vi "PointGrey Grasshopper_Cam_BACKUP.vi"(0 "Operation":T2(ring), 1 "Camera-specific in":variant, 5 "Exposure time (s)":dbl, 7 "Save path":path, 9 "Capture mode":enum16{"Single frame", "Sequence"}(ring), 11 "Capture button":refnum<vi>, 12 "Image in":variant, 14 "Frames in sequence":u32) -> (3 "Camera-specific out":variant, 4 "Status":T1)   [LabVIEW 2015]
uses:
  <vilib>/userdefined/High Color/IMAQdx.ctl
  <vilib>/vision/Image Controls.llb/IMAQ Image.ctl
  <vilib>/vision/driver/IMAQdx.llb/IMAQdx Camera Control Mode.ctl
  <vilib>/vision/driver/IMAQdx.llb/IMAQdx Acquisition Mode.ctl
  <vilib>/Platform/TimedLoop/XDataNode/timing_clust.ctl
  <vilib>/Platform/TimedLoop/XDataNode/nitl_modes.ctl
  <vilib>/Platform/TimedLoop/XDataNode/wakeup.ctl
  <vilib>/vision/driver/IMAQdx.llb/IMAQdx Buffer Number Mode.ctl
  <vilib>/platform/TimedLoop/XDataNode/XDataNode.xnode
  <vilib>/vision/driver/NI_Vision_Acquisition_Software.lvlib
  <resource>/objmgr/imaqdx.rc
  <vilib>/Platform/TimedLoop/XDataNode/XDNodeRunTimeDep.lvlib
  <vilib>/vision/NI_Vision_Development_Module.lvlib
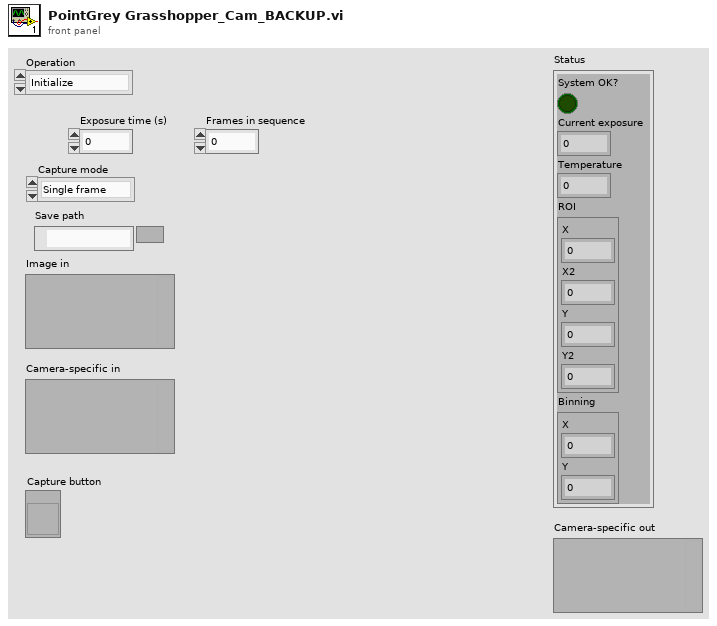
[diagram p1: front panel]
types:
  T1 = cluster{"System OK?":bool, "Current exposure":dbl, "Temperature":dbl, "ROI":cluster{"X":u32, "X2":u32, "Y":u32, "Y2":u32}, "Binning":cluster{"X":u32, "Y":u32}}
  T2 = enum16{"Initialize", "Shut down", "Set capture mode", "Set exposure", "Trigger and read", "Get status", "Other settings"}
  T3 = typedef "IMAQdx.ctl" = refnum<k21>
  T4 = typedef "IMAQ Image.ctl" = refnum<image>
  T5 = typedef "Semaphore RefNum" = refnum<k1>
  T6 = cluster{"Frames to capture":u32, "Current camera":i32, "Camera References":T3[], "Which cameras record":bool[], "Camera event refnums":refnum<event-registration>[], "Image buffers":T4[], "File write access":T5, "Offset and gain":dbl[][], "RGB Channels":enum16{"None", "Camera 1", "Camera 2", "Camera 3"}[], "RGB buffers":T4[], "Camera orientation":enum16{"No rotation, No flip", "No rotation, Flip UD", "No rotation, Flip LR", "Clockwise, No flip", "Clockwise, Flip UD", "Clockwise, Flip LR", "Anticlockwise, No flip", "Anticlockwise, Flip UD", "Anticlockwise, Flip LR"}[]}
  T7 = enum32{"Continuous", "Single frame", "Multi frame"}
  T8 = typedef "NI_Vision_Acquisition_Software.lvlib/IMAQdx Camera Control Mode.ctl" = enum32{"Controller", "Listener"}
  T9 = cluster{"New Image":T4, "Image":refnum<vi>, "FPS target":dbl}
  T10 = enum16{"open", "replace", "create", "open or create", "replace or create", "replace or create with confirmation"}
  T11 = cluster{"File refnum":refnum<file>, "Image File Directory":cluster{cluster{"Field":u16, "Type":u16, "Count":u32, "Value / Offset":u32, "Add IFD Offset?":bool}[], cluster{"Data":u32[], "Add offset?":bool}[]}, "Big endian?":bool, "IFD Offset Size":u32}
  T12 = typedef "NI_Vision_Acquisition_Software.lvlib/IMAQdx Acquisition Mode.ctl" = enum32{"One Shot", "Continuous"}
  T13 = typedef "XDNodeRunTimeDep.lvlib/timing_clust.ctl" = cluster{"Expected End [f-1]":u64, "Actual End [f-1]":u64, "Finished Late? [f-1]":bool, "Expected End [i-1]":u64, "Actual End [i-1]":u64, "Finished Late? [i-1]":bool, "Expected Start [i]":u64, "Actual Start [i]":u64, "Expected Start [f]":u64, "Actual Start [f]":u64, "Source Name":string, "Structure Name":string, "Period":i64, "Deadline":i64, "Offset":i64, "Start":i64, "Priority":i32, "Timeout":i32, "Mode":T14, "Wakeup Reason":T15, "Error":errorcluster, "Source Type":string, "Secondary Source Type":string, "Global End Time":u64, "Global Start Time":u64, "Frame Duration":u64, "Iteration Duration":u64, "Assigned CPU":i32, "I/O Scan Engine Mode":u32}
  T14 = typedef "XDNodeRunTimeDep.lvlib/nitl_modes.ctl" = enum32{"No Change", "Process missed periods, maintain original phase", "Discard missed periods, maintain original phase", "Process missed periods, ignore original phase", "Discard missed periods, ignore original phase"}
  T15 = typedef "XDNodeRunTimeDep.lvlib/wakeup.ctl" = enum32{"Normal", "Aborted", "Asynchronous wakeup", "Timing source error", "Timed loop error", "Timeout"}
  T16 = typedef "NI_Vision_Acquisition_Software.lvlib/IMAQdx Buffer Number Mode.ctl" = enum32{"Next", "Last", "Buffer Number", "Every", "Last New"}
  T17 = enum16{"No rotation, No flip", "No rotation, Flip UD", "No rotation, Flip LR", "Clockwise, No flip", "Clockwise, Flip UD", "Clockwise, Flip LR", "Anticlockwise, No flip", "Anticlockwise, Flip UD", "Anticlockwise, Flip LR"}[]
  T18 = typedef "Image Type" = u32
  T19 = enum16{"None", "Camera 1", "Camera 2", "Camera 3"}[]
  T20 = cluster{"Type":u32, "Version":u32, "Flags":u32, "SerialNumberHigh":u32, "SerialNumberLow":u32, "BusType":u32, "InterfaceName":string, "VendorName":string, "ModelName":string, "CameraFileName":string, "CameraAttributeURL":string}[]
  T21 = enum16{"None", "Camera 1", "Camera 2", "Camera 3"}
  T22 = enum16{"No rotation, No flip", "No rotation, Flip UD", "No rotation, Flip LR", "Clockwise, No flip", "Clockwise, Flip UD", "Clockwise, Flip LR", "Anticlockwise, No flip", "Anticlockwise, Flip UD", "Anticlockwise, Flip LR"}
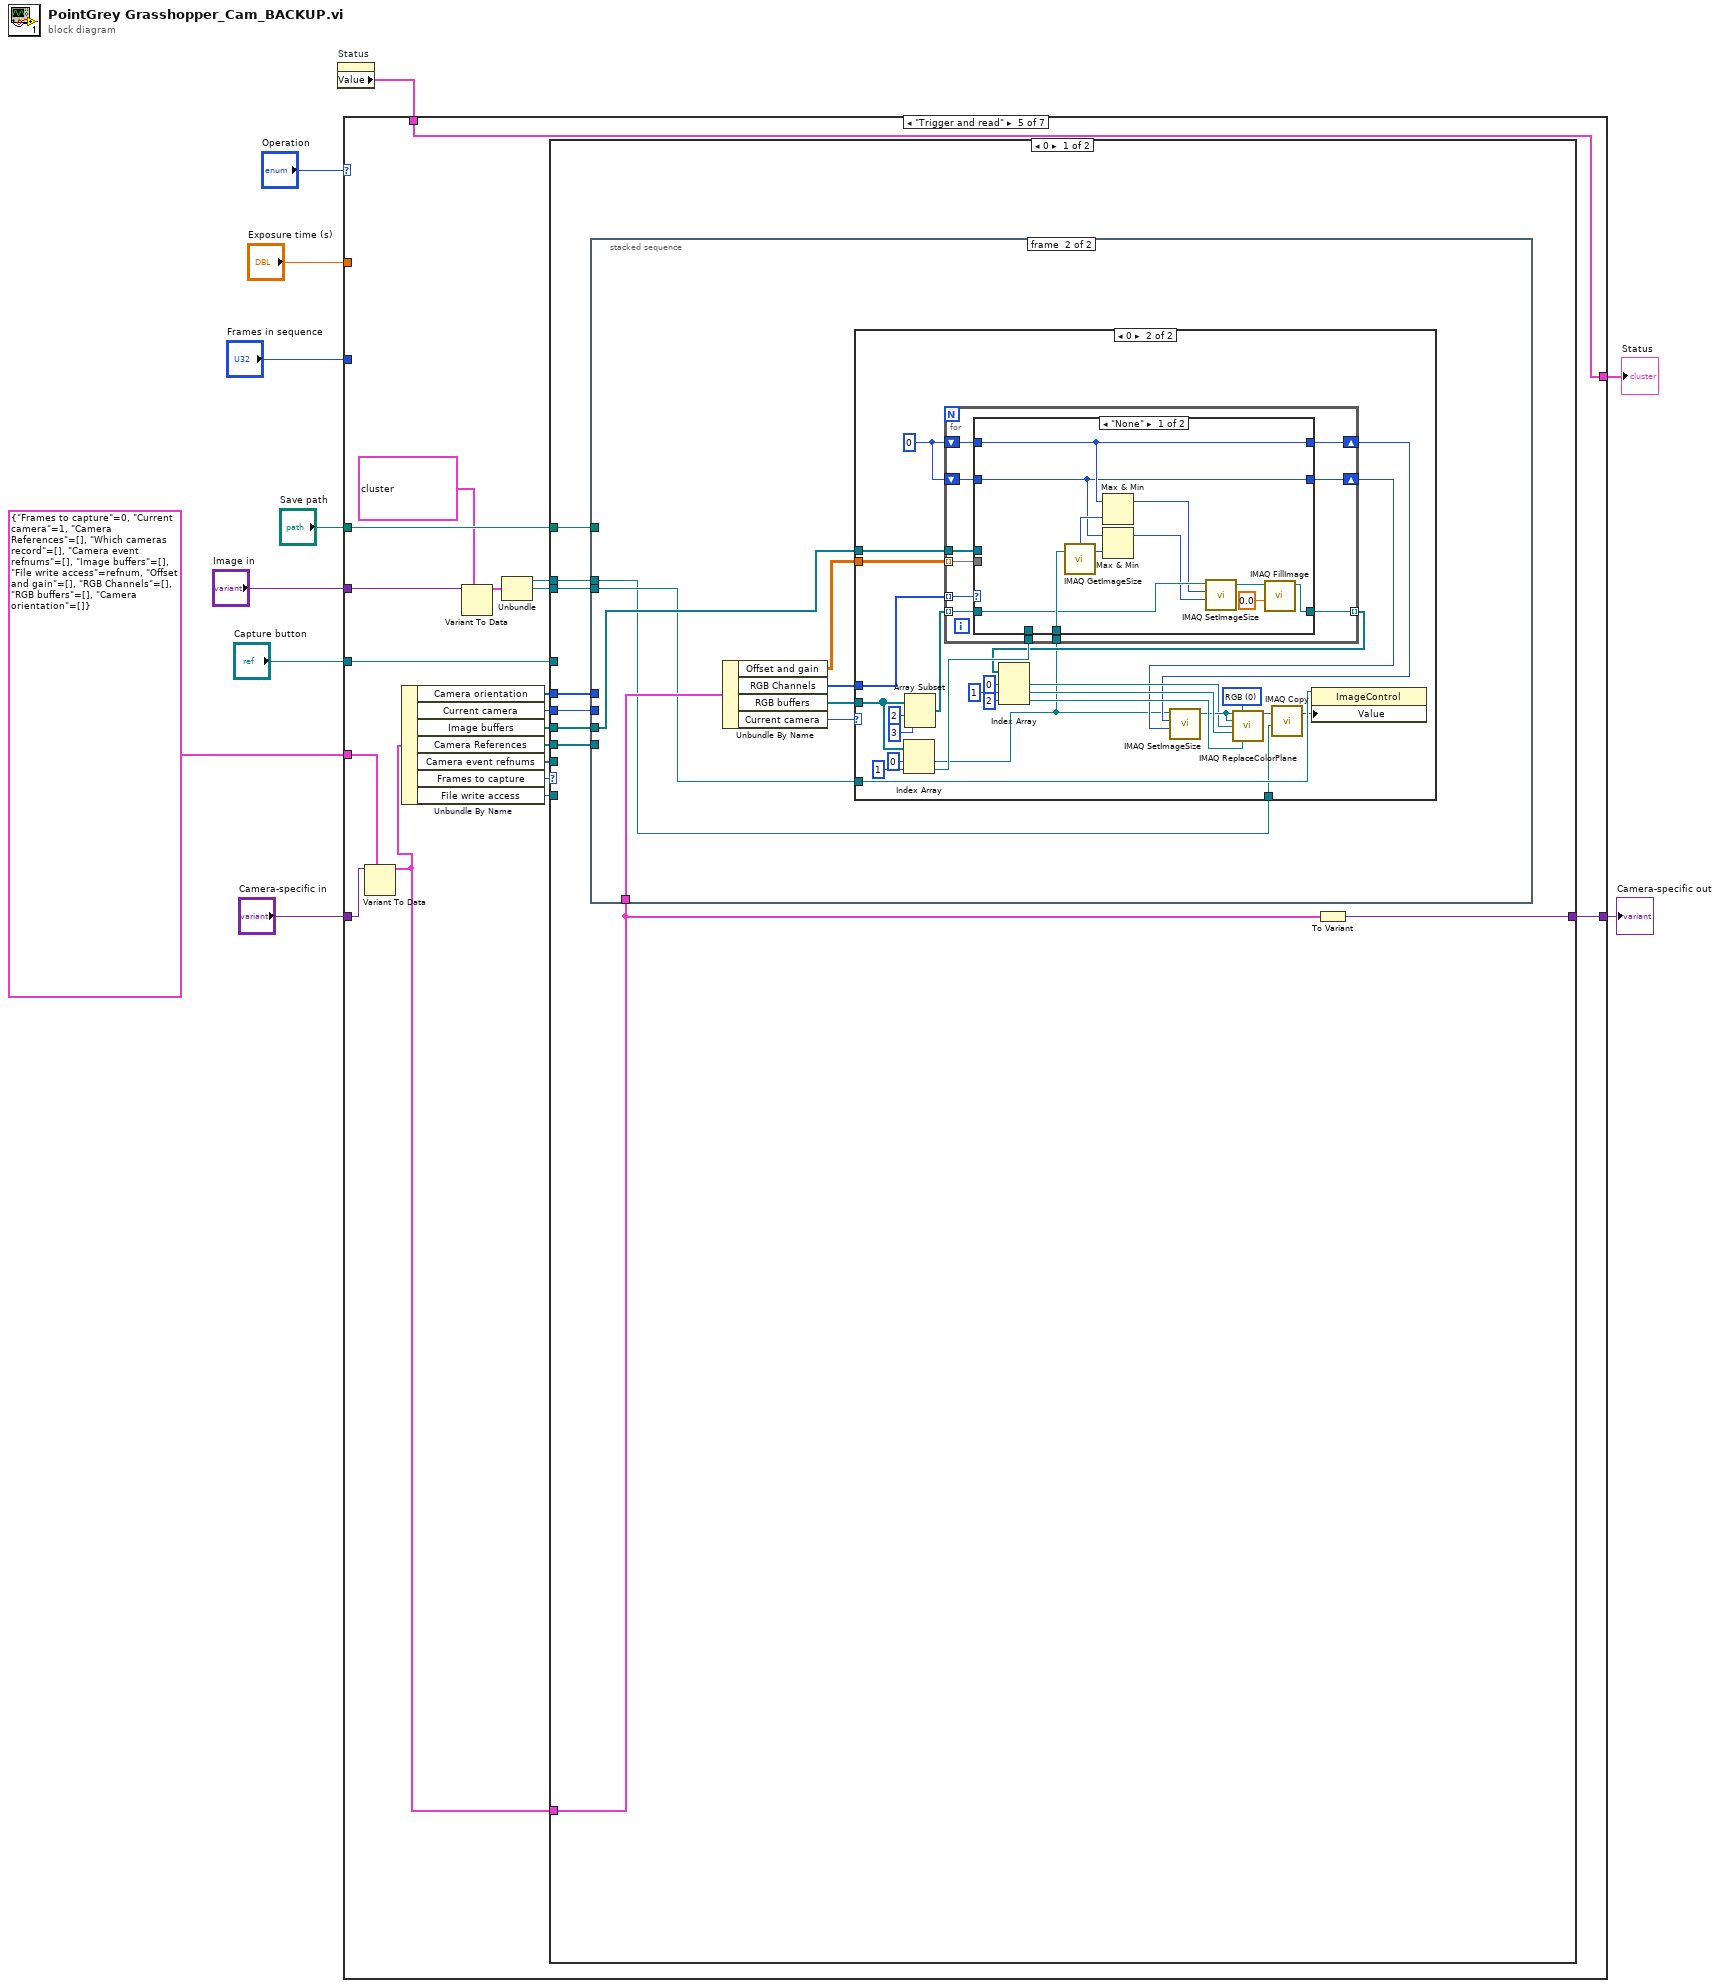
[diagram p0: block diagram]
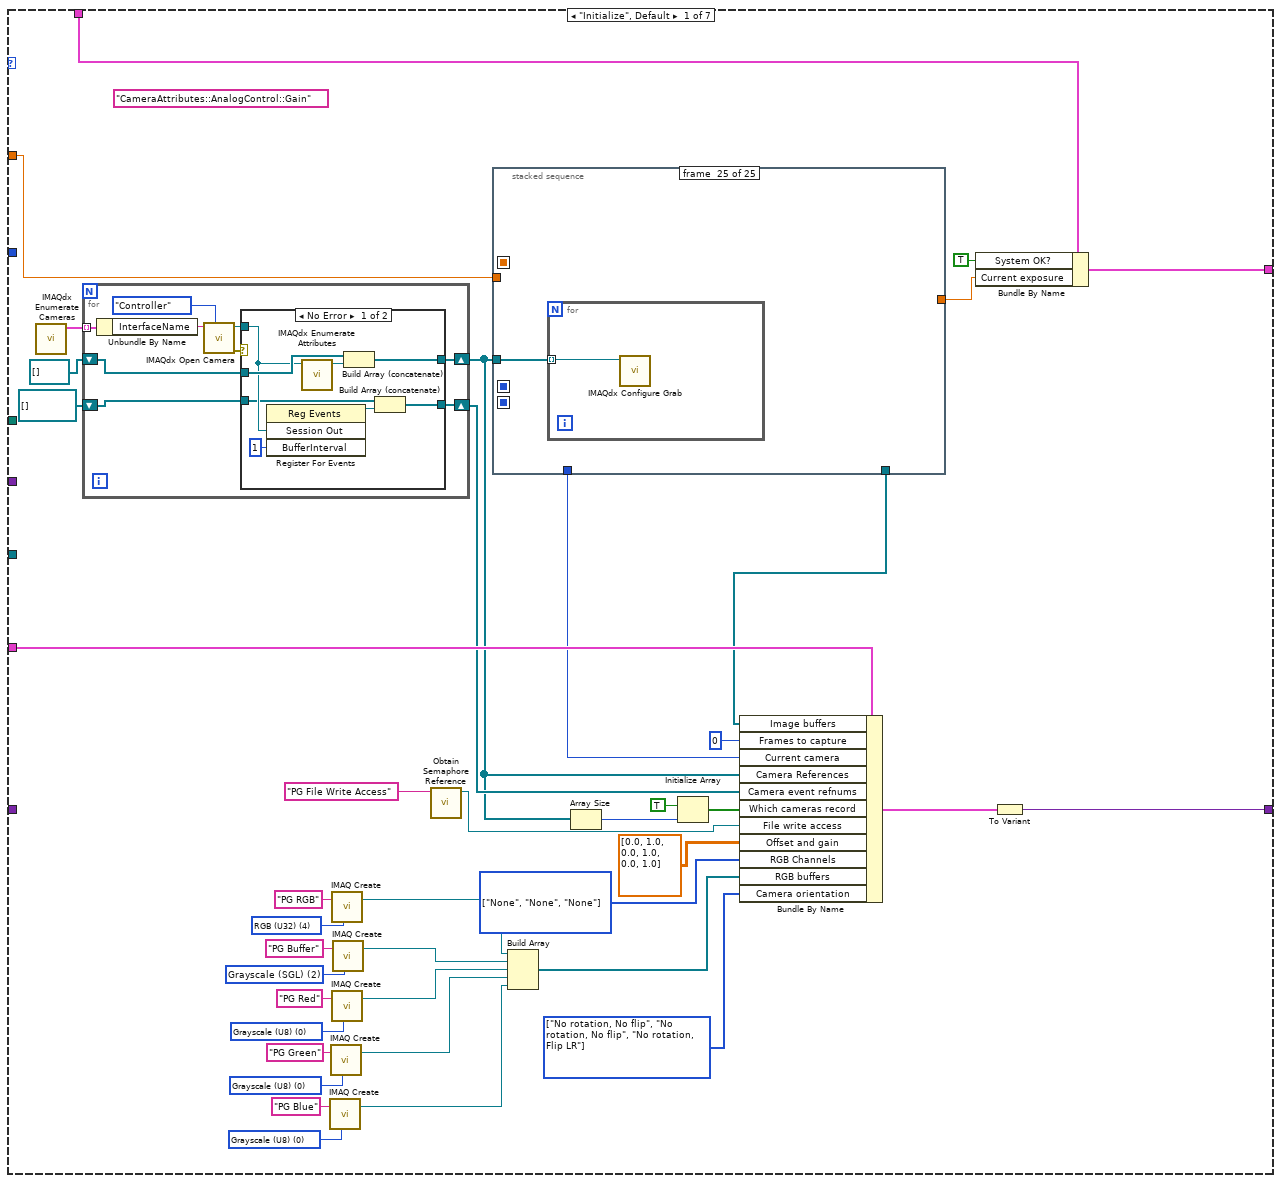
[diagram p2: hidden frame]
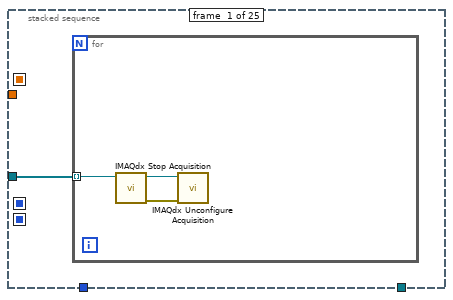
[diagram p3: hidden frame]
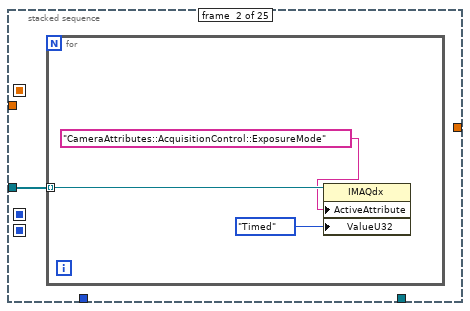
[diagram p4: hidden frame]
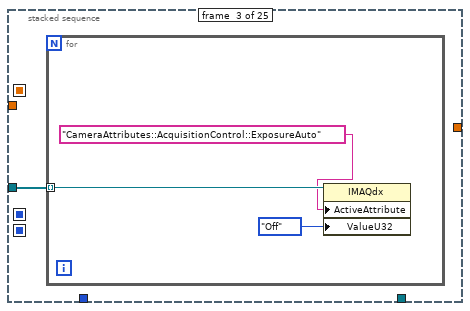
[diagram p5: hidden frame]
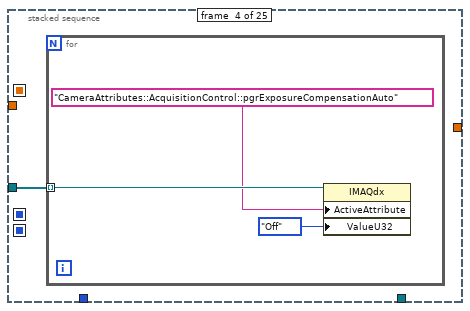
[diagram p6: hidden frame]
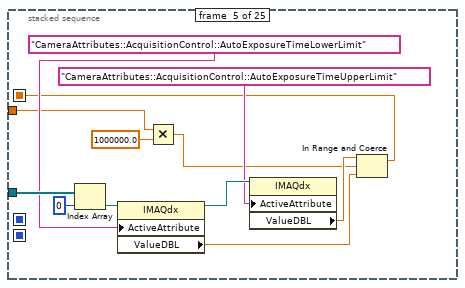
[diagram p7: hidden frame]
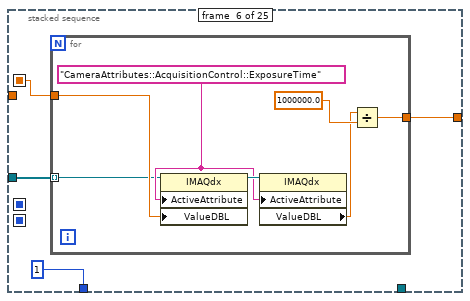
[diagram p8: hidden frame]
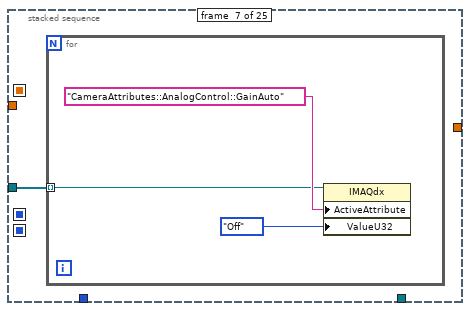
[diagram p9: hidden frame]
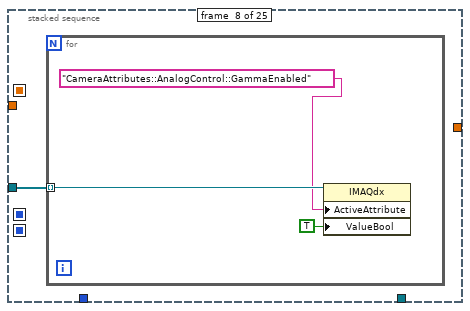
[diagram p10: hidden frame]
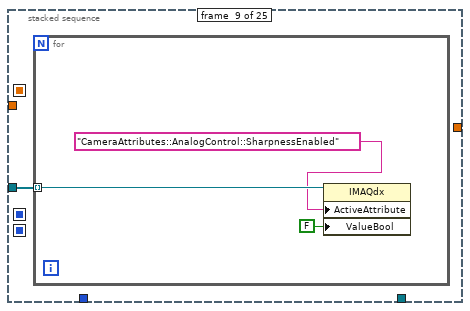
[diagram p11: hidden frame]
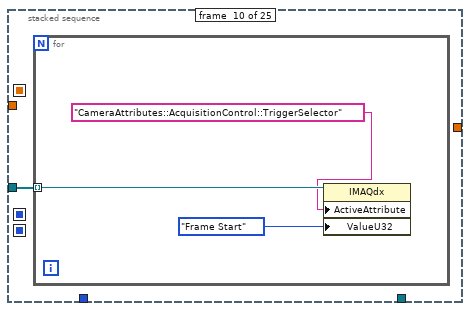
[diagram p12: hidden frame]
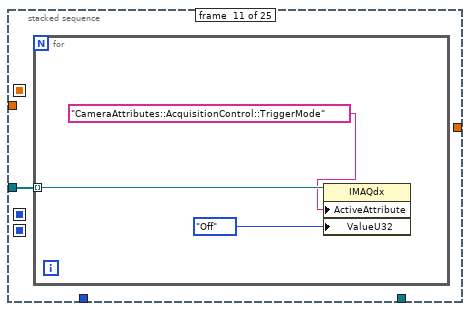
[diagram p13: hidden frame]
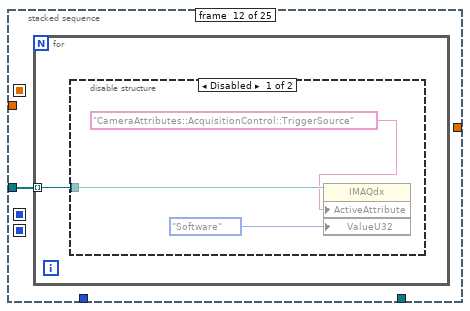
[diagram p14: hidden frame]
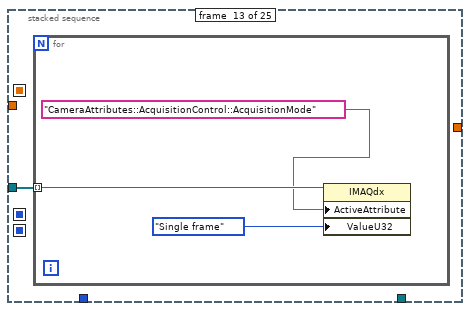
[diagram p16: hidden frame]
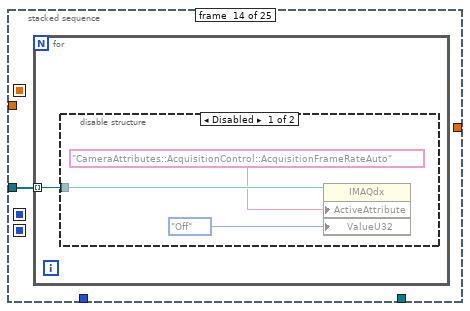
[diagram p17: hidden frame]
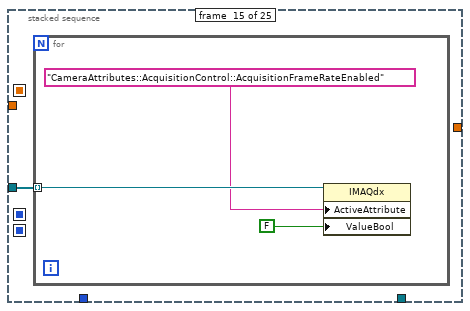
[diagram p19: hidden frame]
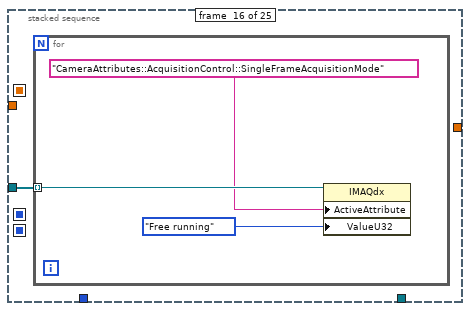
[diagram p20: hidden frame]
diagram:
  n1 = property on="Status" class="Clust (strict)"() -> ("Value"=w9:T1)  [unwired: 2 in, 2 out]
  n2 = case shown="\"Trigger and read\"" "Operation" {
    tunnel: "Exposure time (s)" -> [w40 _ _ w371 _ _ _]
    tunnel: w9 -> [w51 w210 w234 w377 w424 w1366 w1384]
    tunnel: [w50 w210 w234 w376 w424 w1365 w1384] -> w8
    tunnel: "Save path" -> [_ _ _ _ w423 _ _]
    tunnel: "Image in" -> [_ _ _ _ w414 _ _]
    tunnel: [w48 w205 w230 w374 w407 w1362 w1376] -> w5
    tunnel: "Camera-specific in" -> [_ w209 w232 w374 w410 w1362 w1383]
    tunnel: T6 {"Frames to capture"=0, "Current camera"=1, "Camera References"=[], "Which cameras record"=[], "Camera event refnums"=[], "Image buffers"=[], "File write access"=refnum, "Offset and gain"=[], "RGB Channels"=[], "RGB buffers"=[], "Camera orientation"=[]} -> [w49 w204 w231 w375 w422 w1361 w1382]
    tunnel: "Frames in sequence" -> [_ _ w227 _ _ _ _]
    tunnel: "Capture button" -> [_ _ _ _ w406 _ _]
    frame "Initialize", Default {
      w12 = T17 [enum."No rotation, No flip", enum."No rotation, No flip", enum."No rotation, Flip LR"] items=["No rotation, No flip", "No rotation, Flip UD", "No rotation, Flip LR", "Clockwise, No flip", "Clockwise, Flip UD", "Clockwise, Flip LR", "Anticlockwise, No flip", "Anticlockwise, Flip UD", "Anticlockwise, Flip LR"] ("Camera orientation")
      w19 = T18 0 items=["Grayscale (U8)", "Grayscale (I16)", "Grayscale (SGL)", "Complex (CSG)", "RGB (U32)", "HSL (U32)", "RGB (U64)", "Grayscale (U16)"] ("Image Type")
      w20 = T18 0 items=["Grayscale (U8)", "Grayscale (I16)", "Grayscale (SGL)", "Complex (CSG)", "RGB (U32)", "HSL (U32)", "RGB (U64)", "Grayscale (U16)"] ("Image Type")
      w21 = T18 0 items=["Grayscale (U8)", "Grayscale (I16)", "Grayscale (SGL)", "Complex (CSG)", "RGB (U32)", "HSL (U32)", "RGB (U64)", "Grayscale (U16)"] ("Image Type")
      w22 = T18 2 items=["Grayscale (U8)", "Grayscale (I16)", "Grayscale (SGL)", "Complex (CSG)", "RGB (U32)", "HSL (U32)", "RGB (U64)", "Grayscale (U16)"] ("Image Type")
      w23 = T18 4 items=["Grayscale (U8)", "Grayscale (I16)", "Grayscale (SGL)", "Complex (CSG)", "RGB (U32)", "HSL (U32)", "RGB (U64)", "Grayscale (U16)"] ("Image Type")
      w29 = T19 [enum."None", enum."None", enum."None"] items=["None", "Camera 1", "Camera 2", "Camera 3"] ("RGB Channels")
      (unwired) "CameraAttributes::AnalogControl::Gain"
      n3 = call <vilib>:"IMAQdx Enumerate Cameras.vi"() -> ("Camera Information Array"=w46:T20)  [unwired: 10 in, 1 out]
      n4 = for {
        tunnel: w46 -> [w190] mode=indexing
        shift-right: [w185] -> w38
        shift-left: T3[] [] -> [w183]
        shift-right: [w186] -> w43
        shift-left: refnum<event-registration>[] [] -> [w182]
        n5 = Unbundle By Name(w190) -> ("InterfaceName"=w189:string)
        n6 = call <vilib>:"IMAQdx Open Camera.vi"("Camera Control Mode"=IMAQdx_Camera_Control_Mode."Controller", "Session In"=w189) -> ("error out"=w184:errorcluster, "Session Out"=w187:T3)  [unwired: 8 in]
        n7 = case shown="No Error" w184 {
          tunnel: w187 -> [w194 _]
          tunnel: [w193 w199] -> w186
          tunnel: [w196 w200] -> w185
          tunnel: w183 -> [w195 w200]
          tunnel: w182 -> [w191 w199]
          frame No Error {
            n8 = register-events(w194, u32 1 ("BufferInterval")) -> (reference out=w192:refnum<event-registration>)  [unwired: 2 in, 1 out]
            n9 = call <vilib>:"IMAQdx Enumerate Attributes.vi"("Session In"=w194) -> ("Session Out"=w197:T3)  [unwired: 8 in, 2 out]
            n10 = Build Array (concatenate)(w195, w197) -> (w196:T3[])
            n11 = Build Array (concatenate)(w191, w192) -> (w193:refnum<event-registration>[])
          }
          frame Error {
          }
        }
      }
      n12 = call "IMAQ Create"("Image Name"="PG Blue", "Image Type"=w19) -> ("New Image"=w14:T4)  [unwired: 3 in, 1 out]
      n13 = call "IMAQ Create"("Image Name"="PG Green", "Image Type"=w20) -> ("New Image"=w15:T4)  [unwired: 3 in, 1 out]
      n14 = call "IMAQ Create"("Image Name"="PG RGB", "Image Type"=w23) -> ("New Image"=w18:T4)  [unwired: 3 in, 1 out]
      n15 = call "IMAQ Create"("Image Name"="PG Red", "Image Type"=w21) -> ("New Image"=w16:T4)  [unwired: 3 in, 1 out]
      n16 = call "IMAQ Create"("Image Name"="PG Buffer", "Image Type"=w22) -> ("New Image"=w17:T4)  [unwired: 3 in, 1 out]
      n17 = call <vilib>:"Obtain Semaphore Reference.vi"("name (unnamed)"="PG File Write Access") -> ("semaphore"=w31:T5)  [unwired: 4 in, 2 out]
      n18 = stacked-sequence {
        seq-local: [_ _ _ _ w71 _ _ _ _ _ _ _ _ _ _ _ _ _ _ _ _ _ _ _ _] -> [_ _ _ _ _ w80 _ _ _ _ _ _ _ _ _ _ _ _ _ _ _ _ _ _ _]
        seq-local: [_ _ _ _ _ _ _ _ _ _ _ _ _ _ _ _ _ w137 _ _ _ _ _ _ _] -> [_ _ _ _ _ _ _ _ _ _ _ _ _ _ _ _ _ _ _ _ _ _ _ w167 _]
        seq-local: [_ _ _ _ _ _ _ _ _ _ _ _ _ _ _ _ _ _ w143 _ _ _ _ _ _] -> [_ _ _ _ _ _ _ _ _ _ _ _ _ _ _ _ _ _ _ _ _ _ _ w166 _]
        tunnel: w38 -> [w52 w56 w60 w64 w77 w83 w91 w95 w99 w103 w107 w111 w116 w120 w125 w129 w133 w138 w144 w149 w153 w157 w161 w168 w180]
        tunnel: [_ _ _ _ _ 1 ("index") _ _ _ _ _ _ _ _ _ _ _ _ _ _ _ _ _ _ _] -> w41
        tunnel: w40 -> [_ _ _ _ w69 _ _ _ _ _ _ _ _ _ _ _ _ _ _ _ _ _ _ _ _]
        tunnel: [_ _ _ _ _ w81 _ _ _ _ _ _ _ _ _ _ _ _ _ _ _ _ _ _ _] -> w39
        tunnel: [_ _ _ _ _ _ _ _ _ _ _ _ _ _ _ _ _ _ _ _ _ _ _ w165 _] -> w34
        frame #0 {
          n19 = for {
            tunnel: w52 -> [w55] mode=indexing
            n20 = call <vilib>:"IMAQdx Stop Acquisition.vi"("Session In"=w55) -> ("error out"=w53:errorcluster, "Session Out"=w54:T3)  [unwired: 9 in]
            n21 = call <vilib>:"IMAQdx Unconfigure Acquisition.vi"("error in"=w53, "Session In"=w54) -> ()  [unwired: 8 in, 2 out]
          }
        }
        frame #1 {
          n22 = for {
            tunnel: w56 -> [w59] mode=indexing
            n23 = property class="IMAQdx"(reference=w59, "ActiveAttribute"="CameraAttributes::AcquisitionControl::ExposureMode", "ValueU32"=enum32{"Timed", "Trigger Width"}."Timed") -> ()  [unwired: 1 in, 2 out]
          }
        }
        frame #2 {
          n24 = for {
            tunnel: w60 -> [w63] mode=indexing
            n25 = property class="IMAQdx"(reference=w63, "ActiveAttribute"="CameraAttributes::AcquisitionControl::ExposureAuto", "ValueU32"=enum32{"Off", "Once", "Continuous"}."Off") -> ()  [unwired: 1 in, 2 out]
          }
        }
        frame #3 {
          n26 = for {
            tunnel: w64 -> [w67] mode=indexing
            n27 = property class="IMAQdx"(reference=w67, "ActiveAttribute"="CameraAttributes::AcquisitionControl::pgrExposureCompensationAuto", "ValueU32"=enum32{"Off", "Once", "Continuous"}."Off") -> ()  [unwired: 1 in, 2 out]
          }
        }
        frame #4 {
          n28 = Index Array(array=w77, index=0) -> (element=w79:T3)
          n29 = property class="IMAQdx"(reference=w79, "ActiveAttribute"="CameraAttributes::AcquisitionControl::AutoExposureTimeLowerLimit") -> (reference out=w75:T3, "ValueDBL"=w73:dbl)  [unwired: 1 in, 1 out]
          n30 = Multiply(x=w69, y=1000000.0) -> (x*y=w68:dbl)
          n31 = property class="IMAQdx"(reference=w75, "ActiveAttribute"="CameraAttributes::AcquisitionControl::AutoExposureTimeUpperLimit") -> ("ValueDBL"=w72:dbl)  [unwired: 1 in, 2 out]
          n32 = In Range and Coerce(upper limit=w72, x=w68, lower limit=w73) -> (coerced(x)=w71:dbl)  [unwired: 1 out]
        }
        frame #5 {
          n33 = for {
            tunnel: w83 -> [w84] mode=indexing
            tunnel: [w87] -> w81
            tunnel: w80 -> [w85]
            w86 = "CameraAttributes::AcquisitionControl::ExposureTime"
            n34 = property class="IMAQdx"(reference=w84, "ActiveAttribute"=w86, "ValueDBL"=w85) -> (reference out=w90:T3)  [unwired: 1 in, 1 out]
            n35 = property class="IMAQdx"(reference=w90, "ActiveAttribute"=w86) -> ("ValueDBL"=w88:dbl)  [unwired: 1 in, 2 out]
            n36 = Divide(x=w88, y=1000000.0) -> (x/y=w87:dbl)
          }
        }
        frame #6 {
          n37 = for {
            tunnel: w91 -> [w92] mode=indexing
            n38 = property class="IMAQdx"(reference=w92, "ActiveAttribute"="CameraAttributes::AnalogControl::GainAuto", "ValueU32"=enum32{"Off", "Once", "Continuous"}."Off") -> ()  [unwired: 1 in, 2 out]
          }
        }
        frame #7 {
          n39 = for {
            tunnel: w95 -> [w98] mode=indexing
            n40 = property class="IMAQdx"(reference=w98, "ActiveAttribute"="CameraAttributes::AnalogControl::GammaEnabled", "ValueBool"=TRUE) -> ()  [unwired: 1 in, 2 out]
          }
        }
        frame #8 {
          n41 = for {
            tunnel: w99 -> [w102] mode=indexing
            n42 = property class="IMAQdx"(reference=w102, "ActiveAttribute"="CameraAttributes::AnalogControl::SharpnessEnabled", "ValueBool"=FALSE) -> ()  [unwired: 1 in, 2 out]
          }
        }
        frame #9 {
          n43 = for {
            tunnel: w103 -> [w106] mode=indexing
            n44 = property class="IMAQdx"(reference=w106, "ActiveAttribute"="CameraAttributes::AcquisitionControl::TriggerSelector", "ValueU32"=enum32{"Frame Start", "Exposure Active"}."Frame Start") -> ()  [unwired: 1 in, 2 out]
          }
        }
        frame #10 {
          n45 = for {
            tunnel: w107 -> [w110] mode=indexing
            n46 = property class="IMAQdx"(reference=w110, "ActiveAttribute"="CameraAttributes::AcquisitionControl::TriggerMode", "ValueU32"=enum32{"Off", "On"}."Off") -> ()  [unwired: 1 in, 2 out]
          }
        }
        frame #11 {
          n47 = for {
            tunnel: w111 -> [w112] mode=indexing
            n48 = disable-structure shown="Disabled" {
              disable-tunnel: w112 -> [w115 _]
              frame Disabled {
                n49 = property class="IMAQdx"(reference=w115, "ActiveAttribute"="CameraAttributes::AcquisitionControl::TriggerSource", "ValueU32"=enum32{"Software", "Line 0", "Line 2", "Line 3"}."Software") -> ()  [unwired: 1 in, 2 out]
              }
              frame Enabled {
              }
            }
          }
        }
        frame #12 {
          n50 = for {
            tunnel: w116 -> [w119] mode=indexing
            n51 = property class="IMAQdx"(reference=w119, "ActiveAttribute"="CameraAttributes::AcquisitionControl::AcquisitionMode", "ValueU32"=T7."Single frame") -> ()  [unwired: 1 in, 2 out]
          }
        }
        frame #13 {
          n52 = for {
            tunnel: w120 -> [w121] mode=indexing
            n53 = disable-structure shown="Disabled" {
              disable-tunnel: w121 -> [w124 _]
              frame Disabled {
                n54 = property class="IMAQdx"(reference=w124, "ActiveAttribute"="CameraAttributes::AcquisitionControl::AcquisitionFrameRateAuto", "ValueU32"=enum32{"Off", "Continuous"}."Off") -> ()  [unwired: 1 in, 2 out]
              }
              frame Enabled {
              }
            }
          }
        }
        frame #14 {
          n55 = for {
            tunnel: w125 -> [w128] mode=indexing
            n56 = property class="IMAQdx"(reference=w128, "ActiveAttribute"="CameraAttributes::AcquisitionControl::AcquisitionFrameRateEnabled", "ValueBool"=FALSE) -> ()  [unwired: 1 in, 2 out]
          }
        }
        frame #15 {
          n57 = for {
            tunnel: w129 -> [w132] mode=indexing
            n58 = property class="IMAQdx"(reference=w132, "ActiveAttribute"="CameraAttributes::AcquisitionControl::SingleFrameAcquisitionMode", "ValueU32"=enum16{"Free running", "Triggered"}."Free running") -> ()  [unwired: 1 in, 2 out]
          }
        }
        frame #16 {
          n59 = for {
            tunnel: w133 -> [w136] mode=indexing
            w135 = u32 17563654 items=["Mono 8"=17301505, "Mono 12 Packed (IIDC-msb)"=17563654, "Mono 12 Packed"=17563719, "Mono 16"=17825799]
            n60 = property class="IMAQdx"(reference=w136, "ActiveAttribute"="CameraAttributes::ImageFormatControl::PixelFormat", "ValueU32"=w135) -> ()  [unwired: 1 in, 2 out]
          }
        }
        frame #17 {
          n61 = for {
            tunnel: w138 -> [w142] mode=indexing
            tunnel: [w139] -> w137 mode=indexing
            w141 = "CameraAttributes::ImageFormatControl::Width"
            n62 = property class="IMAQdx"(reference=w142, "ActiveAttribute"=w141) -> (reference out=w140:T3, "MaxU32"=w139:u32)  [unwired: 1 in, 1 out]
            n63 = property class="IMAQdx"(reference=w140, "ActiveAttribute"=w141, "ValueU32"=w139) -> ()  [unwired: 1 in, 2 out]
          }
        }
        frame #18 {
          n64 = for {
            tunnel: w144 -> [w148] mode=indexing
            tunnel: [w145] -> w143 mode=indexing
            w147 = "CameraAttributes::ImageFormatControl::Height"
            n65 = property class="IMAQdx"(reference=w148, "ActiveAttribute"=w147) -> (reference out=w146:T3, "MaxU32"=w145:u32)  [unwired: 1 in, 1 out]
            n66 = property class="IMAQdx"(reference=w146, "ActiveAttribute"=w147, "ValueU32"=w145) -> ()  [unwired: 1 in, 2 out]
          }
        }
        frame #19 {
          n67 = for {
            tunnel: w149 -> [w151] mode=indexing
            n68 = property class="IMAQdx"(reference=w151, "ActiveAttribute"="CameraAttributes::ImageFormatControl::OffsetX", "ValueU32"=u32 0) -> ()  [unwired: 1 in, 2 out]
          }
        }
        frame #20 {
          n69 = for {
            tunnel: w153 -> [w155] mode=indexing
            n70 = property class="IMAQdx"(reference=w155, "ActiveAttribute"="CameraAttributes::ImageFormatControl::OffsetY", "ValueU32"=u32 0) -> ()  [unwired: 1 in, 2 out]
          }
        }
        frame #21 {
          n71 = for {
            tunnel: w157 -> [w159] mode=indexing
            n72 = property class="IMAQdx"(reference=w159, "ActiveAttribute"="CameraAttributes::ImageFormatControl::BinningVertical", "ValueU32"=u32 1) -> ()  [unwired: 1 in, 2 out]
          }
        }
        frame #22 {
          n73 = for {
            tunnel: w161 -> [w163] mode=indexing
            w162 = u16 7 items=["Standard"=0, "2x2 Binning"=1, "2x2 Decimation"=2, "High sensitivity 12-bit ADC"=7]
            n74 = property class="IMAQdx"(reference=w163, "ActiveAttribute"="CameraAttributes::ImageFormatControl::VideoMode", "ValueU32"=w162) -> ()  [unwired: 1 in, 2 out]
          }
        }
        frame #23 {
          n75 = for {
            tunnel: w168 -> [_] mode=indexing
            tunnel: w167 -> [w172] mode=indexing
            tunnel: w166 -> [w171] mode=indexing
            tunnel: [w173] -> w165 mode=indexing
            i -> [w177]
            w179 = T18 7 items=["Grayscale (U8)", "Grayscale (I16)", "Grayscale (SGL)", "Complex (CSG)", "RGB (U32)", "HSL (U32)", "RGB (U64)", "Grayscale (U16)"] ("Image Type")
            n76 = Number To Decimal String(number=w177) -> (decimal integer string=w176:string)  [unwired: 1 in]
            n77 = Concatenate Strings("Image ", w176) -> (w175:string)
            n78 = call "IMAQ Create"("Image Name"=w175, "Image Type"=w179) -> ("New Image"=w174:T4)  [unwired: 3 in, 1 out]
            n79 = To Long Integer(number=w172) -> (32bit integer=w170:i32)
            n80 = To Long Integer(number=w171) -> (32bit integer=w169:i32)
            n81 = call "IMAQ SetImageSize"("Y Resolution"=w169, "X Resolution"=w170, "Image"=w174) -> ("Image Out"=w173:T4)  [unwired: 2 in, 1 out]
          }
        }
        frame #24 {
          n82 = for {
            tunnel: w180 -> [w181] mode=indexing
            n83 = call <vilib>:"IMAQdx Configure Grab.vi"("Session In"=w181) -> ()  [unwired: 9 in, 2 out]
          }
        }
      }
      n84 = Build Array(w18, w17, w16, w15, w14) -> (w13:T4[])
      n85 = Array Size(array=w38) -> (size(s)=w36:i32)
      n86 = Initialize Array(TRUE, w36) -> (w35:bool[])
      n87 = Bundle By Name(cluster=w49, "Image buffers"=w34, "Frames to capture"=u32 0, "Current camera"=w41, "Camera References"=w38, "Camera event refnums"=w43, "Which cameras record"=w35, "File write access"=w31, "Offset and gain"=dbl[][] [[0.0, 1.0], [0.0, 1.0], [0.0, 1.0]], "RGB Channels"=w29, "RGB buffers"=w13, "Camera orientation"=w12) -> (w44:T6)
      n88 = Bundle By Name(cluster=w51, "System OK?"=TRUE, "Current exposure"=w39) -> (w50:T1)
      n89 = To Variant(anything=w44) -> (Variant=w48:variant)
    }
    frame "Shut down" {
      n90 = Variant To Data(type=w204, Variant=w209) -> (data=w208:T6)  [unwired: 1 in, 1 out]
      n91 = Unbundle By Name(w208) -> ("Camera References"=w207:T3[], "Camera event refnums"=w206:refnum<event-registration>[], "File write access"=w203:T5, "Image buffers"=w202:T4[], "RGB buffers"=w201:T4[])
      n92 = for {
        tunnel: w202 -> [w212] mode=indexing
        n93 = call "IMAQ Dispose"("Image"=w212) -> ()  [unwired: 5 in, 1 out]
      }
      n94 = for {
        tunnel: w201 -> [w211] mode=indexing
        n95 = call "IMAQ Dispose"("Image"=w211) -> ()  [unwired: 5 in, 1 out]
      }
      n96 = stacked-sequence {
        tunnel: w207 -> [w213 _]
        tunnel: w206 -> [_ w219]
        frame #0 {
          n97 = for {
            tunnel: w213 -> [w214] mode=indexing
            n98 = call <vilib>:"IMAQdx Stop Acquisition.vi"("Session In"=w214) -> ("error out"=w218:errorcluster, "Session Out"=w217:T3)  [unwired: 9 in]
            n99 = call <vilib>:"IMAQdx Unconfigure Acquisition.vi"("error in"=w218, "Session In"=w217) -> ("error out"=w216:errorcluster, "Session Out"=w215:T3)  [unwired: 8 in]
            n100 = call <vilib>:"IMAQdx Close Camera.vi"("error in"=w216, "Session In"=w215) -> ()  [unwired: 9 in, 1 out]
          }
        }
        frame #1 {
          n101 = for {
            tunnel: w219 -> [w221] mode=indexing
            n102 = Unregister For Events(event registration refnum=w221) -> (error out=w220:errorcluster)  [unwired: 1 in]
            n103 = call <vilib>:"Clear Errors.vi"("error in (no error)"=w220) -> ()  [unwired: 5 in, 2 out]
          }
        }
      }
      n104 = call <vilib>:"Release Semaphore Reference.vi"("semaphore"=w203) -> ()  [unwired: 9 in, 2 out]
      n105 = To Variant(anything=w204) -> (Variant=w205:variant)
    }
    frame "Set capture mode" {
      n106 = Variant To Data(type=w231, Variant=w232) -> (data=w226:T6)  [unwired: 1 in, 1 out]
      n107 = Unbundle By Name(w226) -> ("Camera References"=w225:T3[], "Camera event refnums"=w223:refnum<event-registration>[], "Which cameras record"=w224:bool[])
      n108 = case shown="\"Sequence\"" "Capture mode" {
        tunnel: [w235 w302] -> w228
        tunnel: w227 -> [w236 w303]
        tunnel: w225 -> [w240 w307]
        tunnel: w224 -> [w239 w306]
        tunnel: w223 -> [w238 w305]
        tunnel: [w237 w304] -> w222
        frame "Sequence" {
          n109 = stacked-sequence {
            tunnel: w240 -> [_ w249]
            tunnel: w239 -> [_ w248]
            tunnel: w238 -> [w242 w245]
            tunnel: [_ w247] -> w237
            tunnel: w236 -> [w241 w246]
            tunnel: [w241 _] -> w235
            frame #0 {
              n110 = disable-structure shown="Enabled" {
                disable-tunnel: w242 -> [w243 _]
                frame Disabled {
                  n111 = for {
                    tunnel: w243 -> [w244] mode=indexing
                    n112 = Unregister For Events(event registration refnum=w244) -> ()  [unwired: 1 in, 1 out]
                  }
                }
                frame Enabled {
                }
              }
            }
            frame #1 {
              n113 = for {
                tunnel: w249 -> [w254] mode=indexing
                tunnel: w248 -> [w255] mode=indexing
                shift-right: [w253] -> w247
                shift-left: w245 -> [w252]
                tunnel: w246 -> [w251]
                i -> [w250]
                n114 = case shown="True" w255 {
                  tunnel: w254 -> [_ w259]
                  tunnel: [w256 w260] -> w253
                  tunnel: w252 -> [w256 w261]
                  tunnel: w251 -> [_ w258]
                  tunnel: w250 -> [_ w257]
                  frame False {
                  }
                  frame True {
                    n115 = stacked-sequence {
                      tunnel: w261 -> [_ _ _ _ _ _ _ _ w292]
                      tunnel: [_ _ _ _ _ _ _ _ w293] -> w260
                      tunnel: w259 -> [w264 w265 w273 w277 w280 w284 w286 w289 w294]
                      tunnel: w258 -> [_ _ w272 _ _ _ _ _ _]
                      tunnel: w257 -> [_ _ _ _ _ _ _ _ w291]
                      frame #0 {
                        n116 = call <vilib>:"IMAQdx Stop Acquisition.vi"("Session In"=w264) -> ("error out"=w262:errorcluster, "Session Out"=w263:T3)  [unwired: 9 in]
                        n117 = call <vilib>:"IMAQdx Unconfigure Acquisition.vi"("error in"=w262, "Session In"=w263) -> ()  [unwired: 8 in, 2 out]
                      }
                      frame #1 {
                        n118 = disable-structure shown="Enabled" {
                          disable-tunnel: w265 -> [w266 w269]
                          frame Disabled {
                            n119 = property class="IMAQdx"(reference=w266, "ActiveAttribute"="CameraAttributes::AcquisitionControl::AcquisitionMode", "ValueU32"=T7."Multi frame") -> ()  [unwired: 1 in, 2 out]
                          }
                          frame Enabled {
                            n120 = property class="IMAQdx"(reference=w269, "ActiveAttribute"="CameraAttributes::AcquisitionControl::AcquisitionMode", "ValueU32"=T7."Continuous") -> ()  [unwired: 1 in, 2 out]
                          }
                        }
                      }
                      frame #2 {
                        n121 = disable-structure shown="Enabled" {
                          disable-tunnel: w273 -> [w275 _]
                          disable-tunnel: w272 -> [w274 _]
                          frame Disabled {
                            n122 = property class="IMAQdx"(reference=w275, "ActiveAttribute"="CameraAttributes::AcquisitionControl::AcquisitionFrameCount", "ValueU32"=w274) -> ()  [unwired: 1 in, 2 out]
                          }
                          frame Enabled {
                          }
                        }
                      }
                      frame #3 {
                        n123 = property class="IMAQdx"(reference=w277, "ActiveAttribute"="CameraAttributes::AcquisitionControl::TriggerSource", "ValueU32"=enum32{"Software", "Line 0", "Line 2", "Line 3"}."Software") -> ()  [unwired: 1 in, 2 out]
                      }
                      frame #4 {
                        n124 = property class="IMAQdx"(reference=w280, "ActiveAttribute"="CameraAttributes::AcquisitionControl::TriggerSelector", "ValueU32"=enum32{"Frame Start", "Exposure Active"}."Frame Start") -> ()  [unwired: 1 in, 2 out]
                      }
                      frame #5 {
                        n125 = property class="IMAQdx"(reference=w284, "ActiveAttribute"="CameraAttributes::AcquisitionControl::TriggerMode", "ValueU32"=enum32{"Off", "On"}."Off") -> ()  [unwired: 1 in, 2 out]
                      }
                      frame #6 {
                        n126 = property class="IMAQdx"(reference=w286, "ActiveAttribute"="CameraAttributes::AcquisitionControl::SingleFrameAcquisitionMode", "ValueU32"=enum16{"Free running", "Triggered"}."Triggered") -> ()  [unwired: 1 in, 2 out]
                      }
                      frame #7 {
                        n127 = disable-structure shown="Enabled" {
                          disable-tunnel: w289 -> [w290 _]
                          frame Disabled {
                            n128 = call <vilib>:"IMAQdx Configure Grab.vi"("Session In"=w290) -> ()  [unwired: 9 in, 2 out]
                          }
                          frame Enabled {
                          }
                        }
                      }
                      frame #8 {
                        n129 = disable-structure shown="Enabled" {
                          disable-tunnel: w294 -> [w300 _]
                          disable-tunnel: [w298 w301] -> w293
                          disable-tunnel: w292 -> [w297 w301]
                          disable-tunnel: w291 -> [w295 _]
                          frame Disabled {
                            n130 = register-events(w300, u32 1 ("BufferInterval")) -> (reference out=w296:refnum<event-registration>)  [unwired: 2 in, 1 out]
                            n131 = Replace Array Subset(array=w297, new element=w296, index=w295) -> (w298:refnum<event-registration>[])
                          }
                          frame Enabled {
                          }
                        }
                      }
                    }
                  }
                }
              }
            }
          }
        }
        frame "Single frame", Default {
          n132 = stacked-sequence {
            tunnel: w307 -> [_ w316]
            tunnel: w306 -> [_ w315]
            tunnel: w305 -> [w309 w312]
            tunnel: [_ w314] -> w304
            tunnel: w303 -> [_ w313]
            tunnel: [u32 0 ("Frames in sequence") _] -> w302
            frame #0 {
              n133 = disable-structure shown="Enabled" {
                disable-tunnel: w309 -> [w310 _]
                frame Disabled {
                  n134 = for {
                    tunnel: w310 -> [w311] mode=indexing
                    n135 = Unregister For Events(event registration refnum=w311) -> ()  [unwired: 1 in, 1 out]
                  }
                }
                frame Enabled {
                }
              }
            }
            frame #1 {
              n136 = for {
                tunnel: w316 -> [w321] mode=indexing
                tunnel: w315 -> [w322] mode=indexing
                shift-right: [w320] -> w314
                shift-left: w312 -> [w319]
                tunnel: w313 -> [w318]
                i -> [w317]
                n137 = case shown="True" w322 {
                  tunnel: w321 -> [_ w326]
                  tunnel: [w323 w327] -> w320
                  tunnel: w319 -> [w323 w328]
                  tunnel: w318 -> [_ w325]
                  tunnel: w317 -> [_ w324]
                  frame False {
                  }
                  frame True {
                    n138 = stacked-sequence {
                      tunnel: w328 -> [_ w333 _ _ _ _ _ _ _]
                      tunnel: [_ w334 _ _ _ _ _ _ _] -> w327
                      tunnel: w326 -> [w331 w335 w343 w351 w355 w358 w362 w364 w367]
                      tunnel: w325 -> [_ _ _ w350 _ _ _ _ _]
                      tunnel: w324 -> [_ w332 _ _ _ _ _ _ _]
                      frame #0 {
                        n139 = call <vilib>:"IMAQdx Stop Acquisition.vi"("Session In"=w331) -> ("error out"=w329:errorcluster, "Session Out"=w330:T3)  [unwired: 9 in]
                        n140 = call <vilib>:"IMAQdx Unconfigure Acquisition.vi"("error in"=w329, "Session In"=w330) -> ()  [unwired: 8 in, 2 out]
                      }
                      frame #1 {
                        n141 = disable-structure shown="Enabled" {
                          disable-tunnel: w335 -> [w341 _]
                          disable-tunnel: [w339 w342] -> w334
                          disable-tunnel: w333 -> [w338 w342]
                          disable-tunnel: w332 -> [w336 _]
                          frame Disabled {
                            n142 = register-events(w341, u32 1 ("BufferInterval")) -> (reference out=w337:refnum<event-registration>)  [unwired: 2 in, 1 out]
                            n143 = Replace Array Subset(array=w338, new element=w337, index=w336) -> (w339:refnum<event-registration>[])
                          }
                          frame Enabled {
                          }
                        }
                      }
                      frame #2 {
                        n144 = disable-structure shown="Enabled" {
                          disable-tunnel: w343 -> [w344 w347]
                          frame Disabled {
                            n145 = property class="IMAQdx"(reference=w344, "ActiveAttribute"="CameraAttributes::AcquisitionControl::AcquisitionMode", "ValueU32"=T7."Multi frame") -> ()  [unwired: 1 in, 2 out]
                          }
                          frame Enabled {
                            n146 = property class="IMAQdx"(reference=w347, "ActiveAttribute"="CameraAttributes::AcquisitionControl::AcquisitionMode", "ValueU32"=T7."Continuous") -> ()  [unwired: 1 in, 2 out]
                          }
                        }
                      }
                      frame #3 {
                        n147 = disable-structure shown="Enabled" {
                          disable-tunnel: w351 -> [w353 _]
                          disable-tunnel: w350 -> [w352 _]
                          frame Disabled {
                            n148 = property class="IMAQdx"(reference=w353, "ActiveAttribute"="CameraAttributes::AcquisitionControl::AcquisitionFrameCount", "ValueU32"=w352) -> ()  [unwired: 1 in, 2 out]
                          }
                          frame Enabled {
                          }
                        }
                      }
                      frame #4 {
                        n149 = property class="IMAQdx"(reference=w355, "ActiveAttribute"="CameraAttributes::AcquisitionControl::TriggerSource", "ValueU32"=enum32{"Software", "Line 0", "Line 2", "Line 3"}."Software") -> ()  [unwired: 1 in, 2 out]
                      }
                      frame #5 {
                        n150 = property class="IMAQdx"(reference=w358, "ActiveAttribute"="CameraAttributes::AcquisitionControl::TriggerSelector", "ValueU32"=enum32{"Frame Start", "Exposure Active"}."Frame Start") -> ()  [unwired: 1 in, 2 out]
                      }
                      frame #6 {
                        n151 = property class="IMAQdx"(reference=w362, "ActiveAttribute"="CameraAttributes::AcquisitionControl::TriggerMode", "ValueU32"=enum32{"Off", "On"}."Off") -> ()  [unwired: 1 in, 2 out]
                      }
                      frame #7 {
                        n152 = property class="IMAQdx"(reference=w364, "ActiveAttribute"="CameraAttributes::AcquisitionControl::SingleFrameAcquisitionMode", "ValueU32"=enum16{"Free running", "Triggered"}."Triggered") -> ()  [unwired: 1 in, 2 out]
                      }
                      frame #8 {
                        n153 = disable-structure shown="Enabled" {
                          disable-tunnel: w367 -> [w368 _]
                          frame Disabled {
                            n154 = call <vilib>:"IMAQdx Configure Grab.vi"("Session In"=w368) -> ()  [unwired: 9 in, 2 out]
                          }
                          frame Enabled {
                          }
                        }
                      }
                    }
                  }
                }
              }
            }
          }
        }
      }
      n155 = Bundle By Name(cluster=w226, "Frames to capture"=w228, "Camera event refnums"=w222) -> (w229:T6)
      n156 = To Variant(anything=w229) -> (Variant=w230:variant)
    }
    frame "Set exposure" {
      n157 = Variant To Data(type=w375, Variant=w374) -> (data=w373:T6)  [unwired: 1 in, 1 out]
      n158 = Unbundle By Name(w373) -> ("Camera References"=w370:T3[], "Current camera"=w369:i32)
      n159 = case shown="1, Default" w369 {
        selector: w369 -> [_ w380]
        tunnel: [w378 w383] -> w372
        tunnel: w371 -> [w378 w382]
        tunnel: w370 -> [_ w381]
        frame 65535 {
        }
        frame 1, Default {
          n160 = Decrement(x=w380) -> (x-1=w379:i32)
          n161 = stacked-sequence {
            seq-local: [w388 _] -> [_ w397]
            tunnel: w381 -> [w394 w396]
            tunnel: w382 -> [w386 _]
            tunnel: [_ w398] -> w383
            tunnel: w379 -> [_ _]
            frame #0 {
              n162 = Index Array(array=w394, index=0) -> (element=w395:T3)
              n163 = property class="IMAQdx"(reference=w395, "ActiveAttribute"="CameraAttributes::AcquisitionControl::AutoExposureTimeLowerLimit") -> (reference out=w392:T3, "ValueDBL"=w390:dbl)  [unwired: 1 in, 1 out]
              n164 = Multiply(x=w386, y=1000000.0) -> (x*y=w385:dbl)
              n165 = property class="IMAQdx"(reference=w392, "ActiveAttribute"="CameraAttributes::AcquisitionControl::AutoExposureTimeUpperLimit") -> ("ValueDBL"=w389:dbl)  [unwired: 1 in, 2 out]
              n166 = In Range and Coerce(upper limit=w389, x=w385, lower limit=w390) -> (coerced(x)=w388:dbl)  [unwired: 1 out]
            }
            frame #1 {
              n167 = for {
                tunnel: [w402] -> w398
                tunnel: w397 -> [w400]
                tunnel: w396 -> [w399] mode=indexing
                w401 = "CameraAttributes::AcquisitionControl::ExposureTime"
                n168 = property class="IMAQdx"(reference=w399, "ActiveAttribute"=w401, "ValueDBL"=w400) -> (reference out=w405:T3)  [unwired: 1 in, 1 out]
                n169 = property class="IMAQdx"(reference=w405, "ActiveAttribute"=w401) -> ("ValueDBL"=w403:dbl)  [unwired: 1 in, 2 out]
                n170 = Divide(x=w403, y=1000000.0) -> (x/y=w402:dbl)
              }
            }
          }
        }
      }
      n171 = Bundle By Name(cluster=w377, "Current exposure"=w372) -> (w376:T1)
    }
    frame "Trigger and read" {
      n172 = Variant To Data(type=w422, Variant=w410) -> (data=w409:T6)  [unwired: 1 in, 1 out]
      n173 = Unbundle By Name(w409) -> ("Camera orientation"=w408:T17, "Current camera"=w417:i32, "Image buffers"=w418:T4[], "Camera References"=w420:T3[], "Camera event refnums"=w419:refnum<event-registration>[], "Frames to capture"=w421:u32, "File write access"=w411:T5)
      n174 = Variant To Data(type=T9 {"New Image"=refnum, "Image"=refnum, "FPS target"=30.0} ("output cluster"), Variant=w414) -> (data=w416:T9)  [unwired: 1 in, 1 out]
      n175 = Unbundle(w416) -> ("New Image"=w413:T4, "Image"=w412:refnum<vi>)  [unwired: 1 out]
      n176 = case shown="0" w421 {
        selector: w421 -> [_ w617]
        tunnel: w423 -> [w429 w623]
        tunnel: w413 -> [w430 w622]
        tunnel: w420 -> [w433 w621]
        tunnel: w419 -> [_ w620]
        tunnel: w418 -> [w432 w619]
        tunnel: w417 -> [w431 w618]
        tunnel: w412 -> [w428 w616]
        tunnel: w411 -> [_ w615]
        tunnel: w409 -> [w426 w614]
        tunnel: w408 -> [w427 w613]
        tunnel: [w425 w612] -> w407
        tunnel: w406 -> [_ w611]
        frame 0 {
          n177 = stacked-sequence {
            tunnel: w433 -> [w440 _]
            tunnel: w432 -> [w438 w532]
            tunnel: w431 -> [w437 _]
            tunnel: w430 -> [w436 w529]
            tunnel: w429 -> [w435 _]
            tunnel: w426 -> [_ w531]
            tunnel: w428 -> [_ w530]
            tunnel: w427 -> [w434 _]
            frame #0 {
              n178 = Array Size(array=w438) -> (size(s)=w439:i32)
              n179 = for {
                tunnel: w438 -> [w453] mode=indexing
                tunnel: w440 -> [w454] mode=indexing
                workers-P: w439 -> [_]
                tunnel: w437 -> [w452]
                tunnel: w436 -> [w449]
                tunnel: w435 -> [w445]
                tunnel: w434 -> [w441] mode=indexing
                i -> [w451]
                n180 = Decrement(x=w452) -> (x-1=w444:i32)
                n181 = Equal?(x=w444, y=w451) -> (x = y?=w450:bool)
                n182 = call <vilib>:"IMAQdx Snap2.vi"("Image In"=w453, "Session In"=w454) -> ("Image Out"=w443:T4)  [unwired: 7 in, 2 out]
                n183 = case shown="\"Clockwise, Flip LR\"" w441 {
                  tunnel: w443 -> [w455 w458 w461 w464 w471 w478 w481 w490 w497]
                  tunnel: [w455 w457 w460 w462 w467 w474 w482 w486 w493] -> w442
                  frame "No rotation, No flip", Default {
                  }
                  frame "No rotation, Flip UD" {
                    w456 = u32 0 items=["Horizontal", "Vertical", "Central", "1st Diagonal", "2nd Diagonal"] ("Type of Symmetry")
                    n184 = call "IMAQ Symmetry"("Type of Symmetry"=w456, "Image Dst"=w458, "Image Src"=w458) -> ("Image Dst Out"=w457:T4)  [unwired: 2 in, 1 out]
                  }
                  frame "No rotation, Flip LR" {
                    w459 = u32 1 items=["Horizontal", "Vertical", "Central", "1st Diagonal", "2nd Diagonal"] ("Type of Symmetry")
                    n185 = call "IMAQ Symmetry"("Type of Symmetry"=w459, "Image Dst"=w461, "Image Src"=w461) -> ("Image Dst Out"=w460:T4)  [unwired: 2 in, 1 out]
                  }
                  frame "Clockwise, No flip" {
                    n186 = call "IMAQ Rotate"("Use Bilinear Interpolation"=FALSE, "Maintain Size"=FALSE, "Angle (degrees)"=sgl 270.0, "Image Dst"=w464, "Image Src"=w464) -> ("Image Dst Out"=w462:T4)  [unwired: 5 in, 1 out]
                  }
                  frame "Clockwise, Flip UD" {
                    w469 = u32 0 items=["Horizontal", "Vertical", "Central", "1st Diagonal", "2nd Diagonal"] ("Type of Symmetry")
                    n187 = call "IMAQ Rotate"("Use Bilinear Interpolation"=FALSE, "Maintain Size"=FALSE, "Angle (degrees)"=sgl 270.0, "Image Dst"=w471, "Image Src"=w471) -> ("Image Dst Out"=w468:T4)  [unwired: 5 in, 1 out]
                    n188 = call "IMAQ Symmetry"("Type of Symmetry"=w469, "Image Dst"=w468, "Image Src"=w468) -> ("Image Dst Out"=w467:T4)  [unwired: 2 in, 1 out]
                  }
                  frame "Clockwise, Flip LR" {
                    w476 = u32 1 items=["Horizontal", "Vertical", "Central", "1st Diagonal", "2nd Diagonal"] ("Type of Symmetry")
                    n189 = call "IMAQ Rotate"("Use Bilinear Interpolation"=FALSE, "Maintain Size"=FALSE, "Angle (degrees)"=sgl 270.0, "Image Dst"=w478, "Image Src"=w478) -> ("Image Dst Out"=w475:T4)  [unwired: 5 in, 1 out]
                    n190 = call "IMAQ Symmetry"("Type of Symmetry"=w476, "Image Dst"=w475, "Image Src"=w475) -> ("Image Dst Out"=w474:T4)  [unwired: 2 in, 1 out]
                  }
                  frame "Anticlockwise, No flip" {
                    n191 = call "IMAQ Rotate"("Use Bilinear Interpolation"=FALSE, "Maintain Size"=FALSE, "Angle (degrees)"=sgl 90.0, "Image Dst"=w481, "Image Src"=w481) -> ("Image Dst Out"=w482:T4)  [unwired: 5 in, 1 out]
                  }
                  frame "Anticlockwise, Flip UD" {
                    w488 = u32 0 items=["Horizontal", "Vertical", "Central", "1st Diagonal", "2nd Diagonal"] ("Type of Symmetry")
                    n192 = call "IMAQ Rotate"("Use Bilinear Interpolation"=FALSE, "Maintain Size"=FALSE, "Angle (degrees)"=sgl 90.0, "Image Dst"=w490, "Image Src"=w490) -> ("Image Dst Out"=w487:T4)  [unwired: 5 in, 1 out]
                    n193 = call "IMAQ Symmetry"("Type of Symmetry"=w488, "Image Dst"=w487, "Image Src"=w487) -> ("Image Dst Out"=w486:T4)  [unwired: 2 in, 1 out]
                  }
                  frame "Anticlockwise, Flip LR" {
                    w495 = u32 1 items=["Horizontal", "Vertical", "Central", "1st Diagonal", "2nd Diagonal"] ("Type of Symmetry")
                    n194 = call "IMAQ Rotate"("Use Bilinear Interpolation"=FALSE, "Maintain Size"=FALSE, "Angle (degrees)"=sgl 90.0, "Image Dst"=w497, "Image Src"=w497) -> ("Image Dst Out"=w494:T4)  [unwired: 5 in, 1 out]
                    n195 = call "IMAQ Symmetry"("Type of Symmetry"=w495, "Image Dst"=w494, "Image Src"=w494) -> ("Image Dst Out"=w493:T4)  [unwired: 2 in, 1 out]
                  }
                }
                n196 = case shown="True" w450 {
                  tunnel: w442 -> [_ w527]
                  tunnel: w449 -> [_ w528]
                  frame False {
                  }
                  frame True {
                    n197 = call "IMAQ Copy"("Image Dst"=w528, "Image Src"=w527) -> ()  [unwired: 4 in, 2 out]
                  }
                }
                n198 = call "IMAQ GetImageSize"("Image"=w442) -> ("Y Resolution"=w446:i32, "X Resolution"=w447:i32)  [unwired: 3 in, 1 out]
                n199 = Not A Number/Path/Refnum?(number/path/refnum=w445) -> (NaN/Path/Refnum?=w448:bool)
                n200 = case shown="False" w448 {
                  tunnel: w445 -> [w503 _]
                  tunnel: w442 -> [w504 _]
                  tunnel: w447 -> [w501 _]
                  tunnel: w446 -> [w500 _]
                  frame False {
                    n201 = call <vilib>:"Get File Extension.vi"("file"=w503) -> ("lowercase file extension"=w502:string)  [unwired: 6 in, 4 out]
                    n202 = case shown="\"dat\", \"u16\"" w502 {
                      tunnel: w503 -> [w517 w526 _]
                      tunnel: w504 -> [w507 w521 _]
                      tunnel: w501 -> [w515 _ _]
                      tunnel: w500 -> [w514 _ _]
                      frame "'tiff'", "tif" {
                        n203 = call "TIFFStream Open.vi"("Bytes per strip"=u32 8000, "File path"=w517, "Height Pixels"=w514, "Width Pixels"=w515, "Big endian?"=FALSE) -> ("error out"=w511:errorcluster, "Current and next IFD offset"=w509:u32[], "Image data reference"=w508:refnum<data-value>, "File data"=w513:T11)  [unwired: 3 in]
                        n204 = in-place {
                          in-place-border: w507 -> [w519]
                          n205 = in-place-dvr #1(w508) -> ()  [unwired: 2 out]
                          n206 = call "IMAQ ImageToArray"("Image"=w519) -> ("Image Pixels (I16)"=w518:i16[][])  [unwired: 3 in, 4 out]
                          n207 = in-place-dvr #1(w518) -> (w505:refnum<data-value>)  [unwired: 1 out]
                        }
                        n208 = call "TIFFStream Write.vi"("File data"=w513, "error in (no error)"=w511, "Last image in file?"=TRUE, "Current and next IFD offset in"=w509, "Image data reference"=w505) -> ("error out"=w512:errorcluster)  [unwired: 5 in, 1 out]
                        n209 = call "TIFFStream Close.vi"("error in (no error)"=w512, "Image data reference"=w505, "File data"=w513) -> ()  [unwired: 8 in, 1 out]
                      }
                      frame "dat", "u16" {
                        # "No need to cast - no negative values"
                        n210 = Open/Create/Replace File(file path (use dialog)=w526, operation (0:open)=T10."replace or create") -> (refnum out=w525:refnum<file>)  [unwired: 4 in, 2 out]
                        n211 = call "IMAQ ImageToArray"("Image"=w521) -> ("Image Pixels (I16)"=w520:i16[][])  [unwired: 3 in, 4 out]
                        n212 = Write to Binary File(file (use dialog)=w525, data=w520, 5:FALSE ("prepend array or string size? (T)")) -> (refnum out=w523:refnum<file>)  [unwired: 3 in, 2 out]
                        n213 = Close File(refnum=w523) -> ()  [unwired: 1 in, 2 out]
                      }
                      frame "None", Default {
                      }
                    }
                  }
                  frame True {
                  }
                }
              }
            }
            frame #1 {
              n214 = Unbundle By Name(w531) -> ("Offset and gain"=w536:dbl[][], "RGB Channels"=w535:T19, "RGB buffers"=w534:T4[], "Current camera"=w533:i32)
              n215 = case shown="0" w533 {
                tunnel: w536 -> [_ w561]
                tunnel: w535 -> [_ w560]
                tunnel: w532 -> [_ w559]
                tunnel: w534 -> [_ w557]
                tunnel: w530 -> [_ w555]
                tunnel: w529 -> [_ w541]
                frame 1, Default {
                }
                frame 0 {
                  w540 = 0 ("X Resolution")
                  w546 = u16 0 items=["RGB", "HSL", "HSV", "HSI"] ("Color Mode")
                  n216 = Index Array(array=w557, index #1=0 ("index"), index #2=1 ("index")) -> (element #1=w537:T4, element #2=w553:T4)
                  n217 = Array Subset(array=w557, index=2 ("length"), length=3 ("index")) -> (w558:T4[])
                  n218 = for {
                    tunnel: w558 -> [w572] mode=indexing
                    tunnel: w561 -> [w571] mode=indexing
                    tunnel: w560 -> [w574] mode=indexing
                    tunnel: w559 -> [w573]
                    tunnel: [w570] -> w552 mode=indexing
                    tunnel: w553 -> [w569]
                    shift-right: [w565] -> w539
                    shift-left: w540 -> [w568]
                    shift-right: [w566] -> w538
                    shift-left: w540 -> [w567]
                    tunnel: w537 -> [w564]
                    n219 = case shown="\"None\"" w574 {
                      selector: w574 -> [_ w610]
                      tunnel: w573 -> [_ w609]
                      tunnel: w572 -> [w578 w595]
                      tunnel: w571 -> [_ w605]
                      tunnel: [w584 w594] -> w570
                      tunnel: w569 -> [_ w607]
                      tunnel: w568 -> [w582 w590]
                      tunnel: w567 -> [w580 w588]
                      tunnel: [w580 w587] -> w566
                      tunnel: [w582 w586] -> w565
                      tunnel: w564 -> [w583 _]
                      frame "None" {
                        n220 = call "IMAQ GetImageSize"("Image"=w583) -> ("Y Resolution"=w579:i32, "X Resolution"=w581:i32)  [unwired: 3 in, 1 out]
                        n221 = Max & Min(x=w582, y=w581) -> (max(x,y)=w576:i32)  [unwired: 1 out]
                        n222 = Max & Min(x=w580, y=w579) -> (max(x,y)=w575:i32)  [unwired: 1 out]
                        n223 = call "IMAQ SetImageSize"("Y Resolution"=w575, "X Resolution"=w576, "Image"=w578) -> ("Image Out"=w577:T4)  [unwired: 2 in, 1 out]
                        n224 = call "IMAQ FillImage"("Pixel Value (U8, U16, I16, Float)"=sgl 0.0, "Image"=w577) -> ("Image Out"=w584:T4)  [unwired: 8 in, 1 out]
                      }
                      frame "Camera 1", Default {
                        w596 = T18 0 items=["Grayscale (U8)", "Grayscale (I16)", "Grayscale (SGL)", "Complex (CSG)", "RGB (U32)", "HSL (U32)", "RGB (U64)", "Grayscale (U16)"] ("Image Type")
                        w606 = T18 2 items=["Grayscale (U8)", "Grayscale (I16)", "Grayscale (SGL)", "Complex (CSG)", "RGB (U32)", "HSL (U32)", "RGB (U64)", "Grayscale (U16)"] ("Image Type")
                        n225 = Decrement(x=w610) -> (x-1=w608:T21)
                        n226 = Index Array(array=w609, index=w608) -> (element=w593:T4)
                        n227 = call "IMAQ GetImageSize"("Image"=w593) -> ("Y Resolution"=w589:i32, "X Resolution"=w591:i32, "error out"=w592:errorcluster)  [unwired: 3 in]
                        n228 = Index Array(array=w605, index #1=0 ("index"), index #2=1 ("index")) -> (element #1=w602:dbl, element #2=w598:dbl)
                        n229 = call "IMAQ Cast Image"("Image Type"=w606, "error in (no error)"=w592, "Image Dst"=w607, "Image Src"=w593) -> ("Image Dst Out"=w601:T4)  [unwired: 6 in, 1 out]
                        n230 = Max & Min(x=w590, y=w591) -> (max(x,y)=w586:i32)  [unwired: 1 out]
                        n231 = Max & Min(x=w588, y=w589) -> (max(x,y)=w587:i32)  [unwired: 1 out]
                        n232 = call "IMAQ Add"("Image Src A"=w601, "Constant"=w602, "Image Dst"=w601) -> ("Image Dst Out"=w599:T4, "error out"=w600:errorcluster)  [unwired: 4 in]
                        n233 = call "IMAQ Multiply"("Image Src A"=w599, "Constant"=w598, "Image Dst"=w599, "error in (no error)"=w600) -> ("Image Dst Out"=w597:T4)  [unwired: 3 in, 1 out]
                        n234 = call "IMAQ Cast Image"("Image Type"=w596, "Image Dst"=w595, "Image Src"=w597) -> ("Image Dst Out"=w594:T4)  [unwired: 7 in, 1 out]
                      }
                    }
                  }
                  n235 = Index Array(array=w552, index #1=0 ("index"), index #2=1 ("index"), index #3=2 ("index")) -> (element #1=w544:T4, element #2=w548:T4, element #3=w547:T4)
                  n236 = call "IMAQ SetImageSize"("Y Resolution"=w538, "X Resolution"=w539, "Image"=w537) -> ("Image Out"=w545:T4)  [unwired: 2 in, 1 out]
                  n237 = call "IMAQ ReplaceColorPlane"("Image Src"=w545, "Color Mode"=w546, "Image Dst"=w545, "Red or Hue Plane"=w544, "Green or Sat Plane"=w548, "Blue or Luma or Val or Inten Plane"=w547) -> ("Image Dst Out"=w543:T4)  [unwired: 8 in, 1 out]
                  n238 = call "IMAQ Copy"("Image Dst"=w541, "Image Src"=w543) -> ("Image Dst Out"=w542:T4)  [unwired: 4 in, 1 out]
                  n239 = property class="ImageControl"(reference=w555, "Value"=w542) -> ()  [unwired: 1 in, 2 out]
                }
              }
            }
          }
          n240 = To Variant(anything=w426) -> (Variant=w425:variant)
        }
        frame 2, Default {
          n241 = stacked-sequence {
            seq-local: [w641 _ _ _] -> [_ _ w734 w1306]
            seq-local: [w640 _ _ _] -> [_ _ w733 w1305]
            seq-local: [w639 _ _ _] -> [_ _ w732 w1304]
            seq-local: [w638 _ _ _] -> [_ _ w731 w1303]
            seq-local: [w637 _ _ _] -> [_ _ w730 w1300]
            seq-local: [w630 _ _ _] -> [_ _ w712 w1302]
            seq-local: [w624 _ _ _] -> [_ _ w706 _]
            tunnel: w623 -> [w643 _ w729 w1301]
            tunnel: w622 -> [_ _ w713 _]
            tunnel: w621 -> [w625 w696 w736 w1307]
            tunnel: w620 -> [w626 _ _ _]
            tunnel: w619 -> [_ _ w718 _]
            tunnel: w618 -> [_ _ w728 _]
            tunnel: w617 -> [_ _ w709 _]
            tunnel: w616 -> [_ _ w714 _]
            tunnel: w615 -> [_ _ w727 _]
            tunnel: w614 -> [w629 _ w717 _]
            tunnel: w613 -> [_ _ w711 _]
            tunnel: [w628 _ _ _] -> w612
            tunnel: w611 -> [_ _ w705 _]
            frame #0 {
              # "Start acquisition"
              n242 = Index Array(array=w625, index=0) -> (element=w633:T3)
              n243 = for {
                tunnel: w626 -> [w647] mode=indexing
                tunnel: [w645] -> w624 mode=indexing
                tunnel: w625 -> [w646] mode=indexing
                n244 = Unregister For Events(event registration refnum=w647) -> ()  [unwired: 1 in, 1 out]
                n245 = register-events(w646, u32 1 ("BufferInterval")) -> (reference out=w645:refnum<event-registration>)  [unwired: 2 in, 1 out]
              }
              n246 = property class="IMAQdx"(reference=w633, "ActiveAttribute"="CameraAttributes::ImageFormatControl::Width") -> ("ValueU32"=w635:u32)  [unwired: 1 in, 2 out]
              n247 = property class="IMAQdx"(reference=w633, "ActiveAttribute"="CameraAttributes::ImageFormatControl::Height") -> ("ValueU32"=w631:u32)  [unwired: 1 in, 2 out]
              n248 = Not A Number/Path/Refnum?(number/path/refnum=w643) -> (NaN/Path/Refnum?=w642:bool)
              n249 = case shown="False" w642 {
                tunnel: w643 -> [w656 _]
                tunnel: w635 -> [w655 _]
                tunnel: w631 -> [w654 _]
                tunnel: [w653 T11 {"File refnum"=refnum, "Image File Directory"={[], []}, "Big endian?"=FALSE, "IFD Offset Size"=0} ("File data")] -> w639
                tunnel: [w652 refnum<data-value> refnum ("Image data reference")] -> w638
                tunnel: [w651 refnum<queue> refnum ("queue out")] -> w637
                tunnel: [w650 refnum<file> refnum ("refnum out")] -> w640
                tunnel: [w649 "None" ("lowercase file extension")] -> w641
                tunnel: [w648 w691] -> w630
                frame False {
                  n250 = call <vilib>:"Get File Extension.vi"("file"=w656) -> ("lowercase file extension"=w649:string)  [unwired: 6 in, 4 out]
                  n251 = case shown="\"'tiff'\", \"tif\"" w649 {
                    tunnel: w656 -> [w674 w684 _]
                    tunnel: w655 -> [w672 _ _]
                    tunnel: w654 -> [w671 _ _]
                    tunnel: [w669 T11 {"File refnum"=refnum, "Image File Directory"={[], []}, "Big endian?"=FALSE, "IFD Offset Size"=0} ("File data") T11 {"File refnum"=refnum, "Image File Directory"={[], []}, "Big endian?"=FALSE, "IFD Offset Size"=0} ("File data")] -> w653
                    tunnel: [w668 refnum<data-value> refnum ("Image data reference") refnum<data-value> refnum ("Image data reference")] -> w652
                    tunnel: [w661 refnum<queue> refnum ("queue out") refnum<queue> refnum ("queue out")] -> w651
                    tunnel: [refnum<file> refnum ("refnum out") w682 refnum<file> refnum ("refnum out")] -> w650
                    tunnel: [w657 w676 w686] -> w648
                    frame "'tiff'", "tif" {
                      n252 = call "TIFFStream Open.vi"("Bytes per strip"=u32 8000, "File path"=w674, "Height Pixels"=w671, "Width Pixels"=w672, "Big endian?"=FALSE) -> ("Current and next IFD offset"=w663:u32[], "Image data reference"=w668:refnum<data-value>, "File data"=w669:T11)  [unwired: 3 in, 1 out]
                      n253 = Obtain Queue(max queue size (-1, unlimited)=1, name (unnamed)="TIFF position", element data type=w663) -> (queue out=w662:refnum<queue>, error out=w664:errorcluster)  [unwired: 2 in, 1 out]
                      n254 = Lossy Enqueue Element(queue=w662, element=w663, error in (no error)=w664) -> (queue out=w661:refnum<queue>)  [unwired: 3 out]
                      n255 = Obtain Queue(max queue size (-1, unlimited)=-1, name (unnamed)="PG Frame order", element data type=enum16{"Camera 1", "Camera 2", "Camera 3"}."Camera 1" ("Red")) -> (queue out=w657:refnum<queue>)  [unwired: 2 in, 2 out]
                    }
                    frame "dat", "u16" {
                      n256 = Open/Create/Replace File(file path (use dialog)=w684, operation (0:open)=T10."replace or create") -> (refnum out=w682:refnum<file>)  [unwired: 4 in, 2 out]
                      n257 = Obtain Queue(max queue size (-1, unlimited)=-1, name (unnamed)="PG Frame order", element data type=enum16{"Camera 1", "Camera 2", "Camera 3"}."Camera 1" ("Red")) -> (queue out=w676:refnum<queue>)  [unwired: 2 in, 2 out]
                    }
                    frame "None", Default {
                      w686 = refnum<queue> refnum items=["Camera 1", "Camera 2", "Camera 3"] ("queue out")
                    }
                  }
                }
                frame True {
                  w691 = refnum<queue> refnum items=["Camera 1", "Camera 2", "Camera 3"] ("queue out")
                }
              }
              n258 = Bundle By Name(cluster=w629, "Camera event refnums"=w624) -> (w627:T6)
              n259 = To Variant(anything=w627) -> (Variant=w628:variant)
            }
            frame #1 {
              n260 = for {
                tunnel: w696 -> [w697] mode=indexing
                n261 = disable-structure shown="Enabled" {
                  disable-tunnel: w697 -> [w699 w704]
                  frame Disabled {
                    n262 = property class="IMAQdx"(reference=w699, "ActiveAttribute"="CameraAttributes::AcquisitionControl::TriggerSoftware") -> ()  [unwired: 1 in, 2 out]
                  }
                  frame Enabled {
                    n263 = call <vilib>:"IMAQdx Configure Acquisition.vi"("Number of Buffers"=u32 5, "Continuous?"=IMAQdx_Acquisition_Mode."Continuous", "Session In"=w704) -> ("error out"=w700:errorcluster, "Session Out"=w703:T3)  [unwired: 7 in]
                    n264 = call <vilib>:"IMAQdx Start Acquisition.vi"("error in"=w700, "Session In"=w703) -> ()  [unwired: 8 in, 2 out]
                  }
                }
              }
            }
            frame #2 {
              n265 = Obtain Notifier(name (unnamed)="PG Colour", notification data type=FALSE) -> (notifier out=w724:refnum<notifier>, error out=w719:errorcluster)  [unwired: 2 in, 1 out]
              n266 = In Range and Coerce(upper limit=u32 4294967295, x=w709, lower limit=u32 0) -> (coerced(x)=w710:u32)  [unwired: 1 out]
              n267 = Send Notification(notification=FALSE, notifier=w724, error in (no error)=w719) -> (notifier out=w721:refnum<notifier>)  [unwired: 1 out]
              n268 = To Long Integer(number=w710) -> (32bit integer=w735:i32)
              n269 = stacked-sequence {
                tunnel: w706 -> [w847 _]
                tunnel: w736 -> [w835 _]
                tunnel: w718 -> [w834 _]
                tunnel: w735 -> [w820 _]
                tunnel: w734 -> [w805 _]
                tunnel: w733 -> [w806 _]
                tunnel: w732 -> [w807 _]
                tunnel: w731 -> [w808 _]
                tunnel: w730 -> [w818 _]
                tunnel: w729 -> [w815 _]
                tunnel: w728 -> [w813 _]
                tunnel: w713 -> [w812 _]
                tunnel: w714 -> [w811 _]
                tunnel: w727 -> [w810 _]
                tunnel: w721 -> [_ w1299]
                tunnel: w712 -> [w809 _]
                tunnel: w711 -> [w828 _]
                tunnel: w705 -> [w804 _]
                frame #0 {
                  n270 = Index Array(array=w847, index #1=0 ("index"), index #2=1 ("index"), index #3=2 ("index")) -> (element #1=w832:refnum<event-registration>, element #2=w823:refnum<event-registration>, element #3=w814:refnum<event-registration>)
                  n271 = Index Array(array=w828, index #1=0 ("index"), index #2=1 ("index"), index #3=2 ("index")) -> (element #1=w827:T22, element #2=w826:T22, element #3=w819:T22)
                  n272 = Index Array(array=w834, index #1=0 ("index"), index #2=1 ("index"), index #3=2 ("index")) -> (element #1=w840:T4, element #2=w825:T4, element #3=w817:T4)
                  n273 = Index Array(array=w835, index #1=0 ("index"), index #2=1 ("index"), index #3=2 ("index")) -> (element #1=w836:T3, element #2=w824:T3, element #3=w816:T3)
                  n274 = Not A Number/Path/Refnum?(number/path/refnum=w832) -> (NaN/Path/Refnum?=w833:bool)
                  n275 = Not A Number/Path/Refnum?(number/path/refnum=w823) -> (NaN/Path/Refnum?=w822:bool)
                  n276 = Not A Number/Path/Refnum?(number/path/refnum=w814) -> (NaN/Path/Refnum?=w821:bool)
                  n277 = case shown="False" w833 {
                    tunnel: w832 -> [w1164 _]
                    tunnel: w840 -> [w1163 _]
                    tunnel: w836 -> [w1162 _]
                    tunnel: w820 -> [w1161 _]
                    tunnel: w805 -> [w1160 _]
                    tunnel: w806 -> [w1159 _]
                    tunnel: w807 -> [w1158 _]
                    tunnel: w808 -> [w1157 _]
                    tunnel: w818 -> [w1156 _]
                    tunnel: w815 -> [w1155 _]
                    tunnel: w813 -> [w1154 _]
                    tunnel: w812 -> [w1153 _]
                    tunnel: w811 -> [w1152 _]
                    tunnel: w810 -> [w1151 _]
                    tunnel: w809 -> [w1150 _]
                    tunnel: w827 -> [w1149 _]
                    tunnel: w804 -> [w1148 _]
                    frame False {
                      n278 = for {
                        N: w1161 -> [_]
                        tunnel: w1155 -> [w1182]
                        tunnel: w1153 -> [w1181]
                        tunnel: w1164 -> [w1180]
                        tunnel: w1162 -> [w1179]
                        tunnel: w1163 -> [w1178]
                        tunnel: w1154 -> [w1177]
                        tunnel: w1159 -> [w1175]
                        tunnel: w1160 -> [w1174]
                        tunnel: w1158 -> [w1173]
                        tunnel: w1157 -> [w1172]
                        tunnel: w1152 -> [w1171]
                        tunnel: w1156 -> [w1170]
                        tunnel: w1151 -> [w1169]
                        tunnel: w1150 -> [w1168]
                        tunnel: w1149 -> [w1167]
                        tunnel: w1148 -> [w1166]
                        stop <- w1165 stop-if-true
                        n279 = event shown="[1] <Session Out>: Frame Done" {
                          selector: w1180 -> [_ _]
                          dyn-events: _ -> [_ _]
                          timeout: 1000 -> [_ _]
                          tunnel: w1182 -> [_ _]
                          tunnel: w1181 -> [_ w1205]
                          tunnel: w1179 -> [_ w1198]
                          tunnel: w1178 -> [_ w1192]
                          tunnel: w1177 -> [_ w1197]
                          tunnel: w1175 -> [_ w1203]
                          tunnel: w1174 -> [_ w1202]
                          tunnel: w1173 -> [_ w1201]
                          tunnel: w1172 -> [_ w1200]
                          tunnel: w1171 -> [_ w1199]
                          tunnel: w1170 -> [_ w1194]
                          tunnel: w1169 -> [_ w1189]
                          tunnel: w1168 -> [_ w1196]
                          tunnel: w1167 -> [_ w1190]
                          tunnel: w1166 -> [w1185 w1188]
                          tunnel: [w1183 w1186] -> w1165
                          event Timeout {
                            n280 = event-data() -> ()  [unwired: 1 in, 3 out]
                            n281 = property class="Bool (strict)"(reference=w1185) -> ("Value"=w1184:bool)  [unwired: 1 in, 2 out]
                            n282 = Not(x=w1184) -> (.not. x?=w1183:bool)
                          }
                          event event #0x0 {
                            # "Read data"
                            n283 = event-data() -> ()  [unwired: 1 in, 1 out]
                            n284 = Not A Number/Path/Refnum?(number/path/refnum=w1205) -> (NaN/Path/Refnum?=w1206:bool)
                            n285 = call <vilib>:"IMAQdx Get Image2.vi"("Buffer Number Mode (Next)"=IMAQdx_Buffer_Number_Mode."Last New", "Image In"=w1192, "Session In"=w1198) -> ("error out"=w1195:errorcluster, "Image Out"=w1193:T4)  [unwired: 5 in, 2 out]
                            n286 = case shown="\"No rotation, No flip\", Default" w1190 {
                              tunnel: w1193 -> [w1207 w1210 w1213 w1216 w1223 w1230 w1233 w1242 w1249]
                              tunnel: [w1207 w1209 w1212 w1214 w1219 w1226 w1234 w1238 w1245] -> w1191
                              frame "No rotation, No flip", Default {
                              }
                              frame "No rotation, Flip UD" {
                                w1208 = u32 0 items=["Horizontal", "Vertical", "Central", "1st Diagonal", "2nd Diagonal"] ("Type of Symmetry")
                                n287 = call "IMAQ Symmetry"("Type of Symmetry"=w1208, "Image Dst"=w1210, "Image Src"=w1210) -> ("Image Dst Out"=w1209:T4)  [unwired: 2 in, 1 out]
                              }
                              frame "No rotation, Flip LR" {
                                w1211 = u32 1 items=["Horizontal", "Vertical", "Central", "1st Diagonal", "2nd Diagonal"] ("Type of Symmetry")
                                n288 = call "IMAQ Symmetry"("Type of Symmetry"=w1211, "Image Dst"=w1213, "Image Src"=w1213) -> ("Image Dst Out"=w1212:T4)  [unwired: 2 in, 1 out]
                              }
                              frame "Clockwise, No flip" {
                                n289 = call "IMAQ Rotate"("Use Bilinear Interpolation"=FALSE, "Maintain Size"=FALSE, "Angle (degrees)"=sgl 270.0, "Image Dst"=w1216, "Image Src"=w1216) -> ("Image Dst Out"=w1214:T4)  [unwired: 5 in, 1 out]
                              }
                              frame "Clockwise, Flip UD" {
                                w1221 = u32 0 items=["Horizontal", "Vertical", "Central", "1st Diagonal", "2nd Diagonal"] ("Type of Symmetry")
                                n290 = call "IMAQ Rotate"("Use Bilinear Interpolation"=FALSE, "Maintain Size"=FALSE, "Angle (degrees)"=sgl 270.0, "Image Dst"=w1223, "Image Src"=w1223) -> ("Image Dst Out"=w1220:T4)  [unwired: 5 in, 1 out]
                                n291 = call "IMAQ Symmetry"("Type of Symmetry"=w1221, "Image Dst"=w1220, "Image Src"=w1220) -> ("Image Dst Out"=w1219:T4)  [unwired: 2 in, 1 out]
                              }
                              frame "Clockwise, Flip LR" {
                                w1228 = u32 1 items=["Horizontal", "Vertical", "Central", "1st Diagonal", "2nd Diagonal"] ("Type of Symmetry")
                                n292 = call "IMAQ Rotate"("Use Bilinear Interpolation"=FALSE, "Maintain Size"=FALSE, "Angle (degrees)"=sgl 270.0, "Image Dst"=w1230, "Image Src"=w1230) -> ("Image Dst Out"=w1227:T4)  [unwired: 5 in, 1 out]
                                n293 = call "IMAQ Symmetry"("Type of Symmetry"=w1228, "Image Dst"=w1227, "Image Src"=w1227) -> ("Image Dst Out"=w1226:T4)  [unwired: 2 in, 1 out]
                              }
                              frame "Anticlockwise, No flip" {
                                n294 = call "IMAQ Rotate"("Use Bilinear Interpolation"=FALSE, "Maintain Size"=FALSE, "Angle (degrees)"=sgl 90.0, "Image Dst"=w1233, "Image Src"=w1233) -> ("Image Dst Out"=w1234:T4)  [unwired: 5 in, 1 out]
                              }
                              frame "Anticlockwise, Flip UD" {
                                w1240 = u32 0 items=["Horizontal", "Vertical", "Central", "1st Diagonal", "2nd Diagonal"] ("Type of Symmetry")
                                n295 = call "IMAQ Rotate"("Use Bilinear Interpolation"=FALSE, "Maintain Size"=FALSE, "Angle (degrees)"=sgl 90.0, "Image Dst"=w1242, "Image Src"=w1242) -> ("Image Dst Out"=w1239:T4)  [unwired: 5 in, 1 out]
                                n296 = call "IMAQ Symmetry"("Type of Symmetry"=w1240, "Image Dst"=w1239, "Image Src"=w1239) -> ("Image Dst Out"=w1238:T4)  [unwired: 2 in, 1 out]
                              }
                              frame "Anticlockwise, Flip LR" {
                                w1247 = u32 1 items=["Horizontal", "Vertical", "Central", "1st Diagonal", "2nd Diagonal"] ("Type of Symmetry")
                                n297 = call "IMAQ Rotate"("Use Bilinear Interpolation"=FALSE, "Maintain Size"=FALSE, "Angle (degrees)"=sgl 90.0, "Image Dst"=w1249, "Image Src"=w1249) -> ("Image Dst Out"=w1246:T4)  [unwired: 5 in, 1 out]
                                n298 = call "IMAQ Symmetry"("Type of Symmetry"=w1247, "Image Dst"=w1246, "Image Src"=w1246) -> ("Image Dst Out"=w1245:T4)  [unwired: 2 in, 1 out]
                              }
                            }
                            n299 = case shown="False" w1206 {
                              tunnel: w1205 -> [w1289 _]
                              tunnel: w1197 -> [w1290 _]
                              tunnel: w1191 -> [w1288 _]
                              tunnel: w1199 -> [w1287 _]
                              frame False {
                                n300 = case shown="1" w1290 {
                                selector: w1290 -> [_ w1291]
                                tunnel: w1289 -> [_ w1295]
                                tunnel: w1288 -> [_ w1294]
                                tunnel: w1287 -> [_ w1293]
                                frame -1, Default {
                                }
                                frame 1 {
                                n301 = call "IMAQ Copy"("Image Dst"=w1295, "Image Src"=w1294) -> ("Image Dst Out"=w1292:T4)  [unwired: 4 in, 1 out]
                                n302 = case shown="1" w1291 {
                                tunnel: w1293 -> [_ w1297]
                                tunnel: w1292 -> [_ w1296]
                                frame 0, Default {
                                }
                                frame 1 {
                                n303 = property class="ImageControl"(reference=w1297, "Value"=w1296) -> ()  [unwired: 1 in, 2 out]
                                }
                                }
                                }
                                }
                              }
                              frame True {
                              }
                            }
                            n304 = case shown="\"'tiff'\", \"tif\"" w1202 {
                              tunnel: w1191 -> [w1259 _ w1279]
                              tunnel: w1203 -> [_ _ w1278]
                              tunnel: w1201 -> [w1256 _ _]
                              tunnel: w1200 -> [w1257 _ _]
                              tunnel: w1194 -> [w1255 _ _]
                              tunnel: w1189 -> [w1254 _ w1277]
                              tunnel: w1196 -> [w1253 _ w1274]
                              tunnel: w1195 -> [w1252 _ w1276]
                              frame "'tiff'", "tif" {
                                n305 = in-place {
                                in-place-border: w1259 -> [w1273]
                                in-place-border: w1252 -> [w1272]
                                n306 = in-place-dvr #2(w1257) -> ()  [unwired: 2 out]
                                n307 = call "IMAQ ImageToArray"("error in (no error)"=w1272, "Image"=w1273) -> ("Image Pixels (I16)"=w1271:i16[][])  [unwired: 2 in, 4 out]
                                n308 = in-place-dvr #2(w1271) -> (w1258:refnum<data-value>)  [unwired: 1 out]
                                }
                                n309 = stacked-sequence {
                                tunnel: w1258 -> [_ w1267 _ _]
                                tunnel: w1256 -> [_ w1266 _ _]
                                tunnel: w1255 -> [_ w1265 _ _]
                                tunnel: w1254 -> [w1260 _ _ w1270]
                                tunnel: w1253 -> [_ _ w1269 _]
                                frame #0 {
                                n310 = call <vilib>:"Acquire Semaphore.vi"("semaphore"=w1260) -> ()  [unwired: 4 in, 3 out]
                                }
                                frame #1 {
                                n311 = Preview Queue Element(queue=w1265) -> (queue out=w1263:refnum<queue>, element=w1264:u32[])  [unwired: 2 in, 2 out]
                                n312 = call "TIFFStream Write.vi"("File data"=w1266, "Last image in file?"=FALSE, "Current and next IFD offset in"=w1264, "Image data reference"=w1267) -> ("Current and next IFD offset out"=w1262:u32[])  [unwired: 6 in, 1 out]
                                n313 = Lossy Enqueue Element(queue=w1263, element=w1262) -> ()  [unwired: 1 in, 4 out]
                                }
                                frame #2 {
                                n314 = Enqueue Element(queue=w1269, element=enum16{"Camera 1", "Camera 2", "Camera 3"}."Camera 1") -> ()  [unwired: 2 in, 3 out]
                                }
                                frame #3 {
                                n315 = call <vilib>:"Release Semaphore.vi"("semaphore"=w1270) -> ()  [unwired: 5 in, 2 out]
                                }
                                }
                              }
                              frame "None", Default {
                              }
                              frame "dat", "u16" {
                                n316 = call "IMAQ ImageToArray"("error in (no error)"=w1276, "Image"=w1279) -> ("Image Pixels (I16)"=w1275:i16[][])  [unwired: 2 in, 4 out]
                                n317 = stacked-sequence {
                                tunnel: w1275 -> [_ w1282 _ _]
                                tunnel: w1278 -> [_ w1281 _ _]
                                tunnel: w1277 -> [w1280 _ _ w1286]
                                tunnel: w1274 -> [_ _ w1284 _]
                                frame #0 {
                                n318 = call <vilib>:"Acquire Semaphore.vi"("semaphore"=w1280) -> ()  [unwired: 4 in, 3 out]
                                }
                                frame #1 {
                                n319 = Write to Binary File(file (use dialog)=w1281, data=w1282, 5:FALSE ("prepend array or string size? (T)")) -> ()  [unwired: 3 in, 3 out]
                                }
                                frame #2 {
                                n320 = Enqueue Element(queue=w1284, element=enum16{"Camera 1", "Camera 2", "Camera 3"}."Camera 1") -> ()  [unwired: 2 in, 3 out]
                                }
                                frame #3 {
                                n321 = call <vilib>:"Release Semaphore.vi"("semaphore"=w1286) -> ()  [unwired: 5 in, 2 out]
                                }
                                }
                              }
                            }
                            n322 = property class="Bool (strict)"(reference=w1188) -> ("Value"=w1187:bool)  [unwired: 1 in, 2 out]
                            n323 = Not(x=w1187) -> (.not. x?=w1186:bool)
                          }
                        }
                      }
                    }
                    frame True {
                    }
                  }
                  n324 = case shown="False" w822 {
                    tunnel: w823 -> [w1014 _]
                    tunnel: w825 -> [w1013 _]
                    tunnel: w824 -> [w1012 _]
                    tunnel: w820 -> [w1011 _]
                    tunnel: w805 -> [w1010 _]
                    tunnel: w806 -> [w1009 _]
                    tunnel: w807 -> [w1008 _]
                    tunnel: w808 -> [w1007 _]
                    tunnel: w818 -> [w1006 _]
                    tunnel: w815 -> [w1005 _]
                    tunnel: w813 -> [w1004 _]
                    tunnel: w812 -> [w1003 _]
                    tunnel: w811 -> [w1002 _]
                    tunnel: w810 -> [w1001 _]
                    tunnel: w809 -> [w1000 _]
                    tunnel: w826 -> [w999 _]
                    tunnel: w804 -> [w998 _]
                    frame False {
                      n325 = for {
                        N: w1011 -> [_]
                        tunnel: w1005 -> [w1032]
                        tunnel: w1003 -> [w1031]
                        tunnel: w1014 -> [w1030]
                        tunnel: w1012 -> [w1029]
                        tunnel: w1013 -> [w1028]
                        tunnel: w1004 -> [w1027]
                        tunnel: w1009 -> [w1025]
                        tunnel: w1010 -> [w1024]
                        tunnel: w1008 -> [w1023]
                        tunnel: w1007 -> [w1022]
                        tunnel: w1002 -> [w1021]
                        tunnel: w1006 -> [w1020]
                        tunnel: w1001 -> [w1019]
                        tunnel: w1000 -> [w1018]
                        tunnel: w999 -> [w1017]
                        tunnel: w998 -> [w1016]
                        stop <- w1015 stop-if-true
                        n326 = event shown="[1] <Session Out>: Frame Done" {
                          selector: w1030 -> [_ _]
                          dyn-events: _ -> [_ _]
                          timeout: 1000 -> [_ _]
                          tunnel: w1032 -> [_ _]
                          tunnel: w1031 -> [_ w1055]
                          tunnel: w1029 -> [_ w1048]
                          tunnel: w1028 -> [_ w1042]
                          tunnel: w1027 -> [_ w1047]
                          tunnel: w1025 -> [_ w1053]
                          tunnel: w1024 -> [_ w1052]
                          tunnel: w1023 -> [_ w1051]
                          tunnel: w1022 -> [_ w1050]
                          tunnel: w1021 -> [_ w1049]
                          tunnel: w1020 -> [_ w1044]
                          tunnel: w1019 -> [_ w1039]
                          tunnel: w1018 -> [_ w1046]
                          tunnel: w1017 -> [_ w1040]
                          tunnel: w1016 -> [w1035 w1038]
                          tunnel: [w1033 w1036] -> w1015
                          event Timeout {
                            n327 = event-data() -> ()  [unwired: 1 in, 3 out]
                            n328 = property class="Bool (strict)"(reference=w1035) -> ("Value"=w1034:bool)  [unwired: 1 in, 2 out]
                            n329 = Not(x=w1034) -> (.not. x?=w1033:bool)
                          }
                          event event #0x0 {
                            # "Read data"
                            n330 = event-data() -> ()  [unwired: 1 in, 1 out]
                            n331 = Not A Number/Path/Refnum?(number/path/refnum=w1055) -> (NaN/Path/Refnum?=w1056:bool)
                            n332 = call <vilib>:"IMAQdx Get Image2.vi"("Buffer Number Mode (Next)"=IMAQdx_Buffer_Number_Mode."Last New", "Image In"=w1042, "Session In"=w1048) -> ("error out"=w1045:errorcluster, "Image Out"=w1043:T4)  [unwired: 5 in, 2 out]
                            n333 = case shown="\"Anticlockwise, Flip UD\"" w1040 {
                              tunnel: w1043 -> [w1057 w1060 w1063 w1066 w1073 w1080 w1083 w1092 w1099]
                              tunnel: [w1057 w1059 w1062 w1064 w1069 w1076 w1084 w1088 w1095] -> w1041
                              frame "No rotation, No flip", Default {
                              }
                              frame "No rotation, Flip UD" {
                                w1058 = u32 0 items=["Horizontal", "Vertical", "Central", "1st Diagonal", "2nd Diagonal"] ("Type of Symmetry")
                                n334 = call "IMAQ Symmetry"("Type of Symmetry"=w1058, "Image Dst"=w1060, "Image Src"=w1060) -> ("Image Dst Out"=w1059:T4)  [unwired: 2 in, 1 out]
                              }
                              frame "No rotation, Flip LR" {
                                w1061 = u32 1 items=["Horizontal", "Vertical", "Central", "1st Diagonal", "2nd Diagonal"] ("Type of Symmetry")
                                n335 = call "IMAQ Symmetry"("Type of Symmetry"=w1061, "Image Dst"=w1063, "Image Src"=w1063) -> ("Image Dst Out"=w1062:T4)  [unwired: 2 in, 1 out]
                              }
                              frame "Clockwise, No flip" {
                                n336 = call "IMAQ Rotate"("Use Bilinear Interpolation"=FALSE, "Maintain Size"=FALSE, "Angle (degrees)"=sgl 270.0, "Image Dst"=w1066, "Image Src"=w1066) -> ("Image Dst Out"=w1064:T4)  [unwired: 5 in, 1 out]
                              }
                              frame "Clockwise, Flip UD" {
                                w1071 = u32 0 items=["Horizontal", "Vertical", "Central", "1st Diagonal", "2nd Diagonal"] ("Type of Symmetry")
                                n337 = call "IMAQ Rotate"("Use Bilinear Interpolation"=FALSE, "Maintain Size"=FALSE, "Angle (degrees)"=sgl 270.0, "Image Dst"=w1073, "Image Src"=w1073) -> ("Image Dst Out"=w1070:T4)  [unwired: 5 in, 1 out]
                                n338 = call "IMAQ Symmetry"("Type of Symmetry"=w1071, "Image Dst"=w1070, "Image Src"=w1070) -> ("Image Dst Out"=w1069:T4)  [unwired: 2 in, 1 out]
                              }
                              frame "Clockwise, Flip LR" {
                                w1078 = u32 1 items=["Horizontal", "Vertical", "Central", "1st Diagonal", "2nd Diagonal"] ("Type of Symmetry")
                                n339 = call "IMAQ Rotate"("Use Bilinear Interpolation"=FALSE, "Maintain Size"=FALSE, "Angle (degrees)"=sgl 270.0, "Image Dst"=w1080, "Image Src"=w1080) -> ("Image Dst Out"=w1077:T4)  [unwired: 5 in, 1 out]
                                n340 = call "IMAQ Symmetry"("Type of Symmetry"=w1078, "Image Dst"=w1077, "Image Src"=w1077) -> ("Image Dst Out"=w1076:T4)  [unwired: 2 in, 1 out]
                              }
                              frame "Anticlockwise, No flip" {
                                n341 = call "IMAQ Rotate"("Use Bilinear Interpolation"=FALSE, "Maintain Size"=FALSE, "Angle (degrees)"=sgl 90.0, "Image Dst"=w1083, "Image Src"=w1083) -> ("Image Dst Out"=w1084:T4)  [unwired: 5 in, 1 out]
                              }
                              frame "Anticlockwise, Flip UD" {
                                w1090 = u32 0 items=["Horizontal", "Vertical", "Central", "1st Diagonal", "2nd Diagonal"] ("Type of Symmetry")
                                n342 = call "IMAQ Rotate"("Use Bilinear Interpolation"=FALSE, "Maintain Size"=FALSE, "Angle (degrees)"=sgl 90.0, "Image Dst"=w1092, "Image Src"=w1092) -> ("Image Dst Out"=w1089:T4)  [unwired: 5 in, 1 out]
                                n343 = call "IMAQ Symmetry"("Type of Symmetry"=w1090, "Image Dst"=w1089, "Image Src"=w1089) -> ("Image Dst Out"=w1088:T4)  [unwired: 2 in, 1 out]
                              }
                              frame "Anticlockwise, Flip LR" {
                                w1097 = u32 1 items=["Horizontal", "Vertical", "Central", "1st Diagonal", "2nd Diagonal"] ("Type of Symmetry")
                                n344 = call "IMAQ Rotate"("Use Bilinear Interpolation"=FALSE, "Maintain Size"=FALSE, "Angle (degrees)"=sgl 90.0, "Image Dst"=w1099, "Image Src"=w1099) -> ("Image Dst Out"=w1096:T4)  [unwired: 5 in, 1 out]
                                n345 = call "IMAQ Symmetry"("Type of Symmetry"=w1097, "Image Dst"=w1096, "Image Src"=w1096) -> ("Image Dst Out"=w1095:T4)  [unwired: 2 in, 1 out]
                              }
                            }
                            n346 = case shown="False" w1056 {
                              tunnel: w1055 -> [w1139 _]
                              tunnel: w1047 -> [w1140 _]
                              tunnel: w1041 -> [w1138 _]
                              tunnel: w1049 -> [w1137 _]
                              frame False {
                                n347 = case shown="2" w1140 {
                                selector: w1140 -> [_ w1141]
                                tunnel: w1139 -> [_ w1145]
                                tunnel: w1138 -> [_ w1144]
                                tunnel: w1137 -> [_ w1143]
                                frame -1, Default {
                                }
                                frame 2 {
                                n348 = call "IMAQ Copy"("Image Dst"=w1145, "Image Src"=w1144) -> ("Image Dst Out"=w1142:T4)  [unwired: 4 in, 1 out]
                                n349 = case shown="2" w1141 {
                                tunnel: w1143 -> [_ w1147]
                                tunnel: w1142 -> [_ w1146]
                                frame 0, Default {
                                }
                                frame 2 {
                                n350 = property class="ImageControl"(reference=w1147, "Value"=w1146) -> ()  [unwired: 1 in, 2 out]
                                }
                                }
                                }
                                }
                              }
                              frame True {
                              }
                            }
                            n351 = case shown="\"'tiff'\", \"tif\"" w1052 {
                              tunnel: w1041 -> [w1109 _ w1129]
                              tunnel: w1053 -> [_ _ w1128]
                              tunnel: w1051 -> [w1106 _ _]
                              tunnel: w1050 -> [w1107 _ _]
                              tunnel: w1044 -> [w1105 _ _]
                              tunnel: w1039 -> [w1104 _ w1127]
                              tunnel: w1046 -> [w1103 _ w1124]
                              tunnel: w1045 -> [w1102 _ w1126]
                              frame "'tiff'", "tif" {
                                n352 = in-place {
                                in-place-border: w1109 -> [w1123]
                                in-place-border: w1102 -> [w1122]
                                n353 = in-place-dvr #3(w1107) -> ()  [unwired: 2 out]
                                n354 = call "IMAQ ImageToArray"("error in (no error)"=w1122, "Image"=w1123) -> ("Image Pixels (I16)"=w1121:i16[][])  [unwired: 2 in, 4 out]
                                n355 = in-place-dvr #3(w1121) -> (w1108:refnum<data-value>)  [unwired: 1 out]
                                }
                                n356 = stacked-sequence {
                                tunnel: w1108 -> [_ w1117 _ _]
                                tunnel: w1106 -> [_ w1116 _ _]
                                tunnel: w1105 -> [_ w1115 _ _]
                                tunnel: w1104 -> [w1110 _ _ w1120]
                                tunnel: w1103 -> [_ _ w1119 _]
                                frame #0 {
                                n357 = call <vilib>:"Acquire Semaphore.vi"("semaphore"=w1110) -> ()  [unwired: 4 in, 3 out]
                                }
                                frame #1 {
                                n358 = Preview Queue Element(queue=w1115) -> (queue out=w1113:refnum<queue>, element=w1114:u32[])  [unwired: 2 in, 2 out]
                                n359 = call "TIFFStream Write.vi"("File data"=w1116, "Last image in file?"=FALSE, "Current and next IFD offset in"=w1114, "Image data reference"=w1117) -> ("Current and next IFD offset out"=w1112:u32[])  [unwired: 6 in, 1 out]
                                n360 = Lossy Enqueue Element(queue=w1113, element=w1112) -> ()  [unwired: 1 in, 4 out]
                                }
                                frame #2 {
                                n361 = Enqueue Element(queue=w1119, element=enum16{"Camera 1", "Camera 2", "Camera 3"}."Camera 2") -> ()  [unwired: 2 in, 3 out]
                                }
                                frame #3 {
                                n362 = call <vilib>:"Release Semaphore.vi"("semaphore"=w1120) -> ()  [unwired: 5 in, 2 out]
                                }
                                }
                              }
                              frame "None", Default {
                              }
                              frame "dat", "u16" {
                                n363 = call "IMAQ ImageToArray"("error in (no error)"=w1126, "Image"=w1129) -> ("Image Pixels (I16)"=w1125:i16[][])  [unwired: 2 in, 4 out]
                                n364 = stacked-sequence {
                                tunnel: w1125 -> [_ w1132 _ _]
                                tunnel: w1128 -> [_ w1131 _ _]
                                tunnel: w1127 -> [w1130 _ _ w1136]
                                tunnel: w1124 -> [_ _ w1134 _]
                                frame #0 {
                                n365 = call <vilib>:"Acquire Semaphore.vi"("semaphore"=w1130) -> ()  [unwired: 4 in, 3 out]
                                }
                                frame #1 {
                                n366 = Write to Binary File(file (use dialog)=w1131, data=w1132, 5:FALSE ("prepend array or string size? (T)")) -> ()  [unwired: 3 in, 3 out]
                                }
                                frame #2 {
                                n367 = Enqueue Element(queue=w1134, element=enum16{"Camera 1", "Camera 2", "Camera 3"}."Camera 2") -> ()  [unwired: 2 in, 3 out]
                                }
                                frame #3 {
                                n368 = call <vilib>:"Release Semaphore.vi"("semaphore"=w1136) -> ()  [unwired: 5 in, 2 out]
                                }
                                }
                              }
                            }
                            n369 = property class="Bool (strict)"(reference=w1038) -> ("Value"=w1037:bool)  [unwired: 1 in, 2 out]
                            n370 = Not(x=w1037) -> (.not. x?=w1036:bool)
                          }
                        }
                      }
                    }
                    frame True {
                    }
                  }
                  n371 = case shown="False" w821 {
                    tunnel: w814 -> [w864 _]
                    tunnel: w817 -> [w863 _]
                    tunnel: w816 -> [w862 _]
                    tunnel: w820 -> [w861 _]
                    tunnel: w805 -> [w860 _]
                    tunnel: w806 -> [w859 _]
                    tunnel: w807 -> [w858 _]
                    tunnel: w808 -> [w857 _]
                    tunnel: w818 -> [w856 _]
                    tunnel: w815 -> [w855 _]
                    tunnel: w813 -> [w854 _]
                    tunnel: w812 -> [w853 _]
                    tunnel: w811 -> [w852 _]
                    tunnel: w810 -> [w851 _]
                    tunnel: w809 -> [w850 _]
                    tunnel: w819 -> [w849 _]
                    tunnel: w804 -> [w848 _]
                    frame False {
                      n372 = for {
                        N: w861 -> [_]
                        tunnel: w855 -> [w882]
                        tunnel: w853 -> [w881]
                        tunnel: w864 -> [w880]
                        tunnel: w862 -> [w879]
                        tunnel: w863 -> [w878]
                        tunnel: w854 -> [w877]
                        tunnel: w859 -> [w875]
                        tunnel: w860 -> [w874]
                        tunnel: w858 -> [w873]
                        tunnel: w857 -> [w872]
                        tunnel: w852 -> [w871]
                        tunnel: w856 -> [w870]
                        tunnel: w851 -> [w869]
                        tunnel: w850 -> [w868]
                        tunnel: w849 -> [w867]
                        tunnel: w848 -> [w866]
                        stop <- w865 stop-if-true
                        n373 = event shown="[1] <Session Out>: Frame Done" {
                          selector: w880 -> [_ _]
                          dyn-events: _ -> [_ _]
                          timeout: 1000 -> [_ _]
                          tunnel: w882 -> [_ _]
                          tunnel: w881 -> [_ w905]
                          tunnel: w879 -> [_ w898]
                          tunnel: w878 -> [_ w892]
                          tunnel: w877 -> [_ w897]
                          tunnel: w875 -> [_ w903]
                          tunnel: w874 -> [_ w902]
                          tunnel: w873 -> [_ w901]
                          tunnel: w872 -> [_ w900]
                          tunnel: w871 -> [_ w899]
                          tunnel: w870 -> [_ w894]
                          tunnel: w869 -> [_ w889]
                          tunnel: w868 -> [_ w896]
                          tunnel: w867 -> [_ w890]
                          tunnel: w866 -> [w885 w888]
                          tunnel: [w883 w886] -> w865
                          event Timeout {
                            n374 = event-data() -> ()  [unwired: 1 in, 3 out]
                            n375 = property class="Bool (strict)"(reference=w885) -> ("Value"=w884:bool)  [unwired: 1 in, 2 out]
                            n376 = Not(x=w884) -> (.not. x?=w883:bool)
                          }
                          event event #0x0 {
                            # "Read data"
                            n377 = event-data() -> ()  [unwired: 1 in, 1 out]
                            n378 = Not A Number/Path/Refnum?(number/path/refnum=w905) -> (NaN/Path/Refnum?=w906:bool)
                            n379 = call <vilib>:"IMAQdx Get Image2.vi"("Buffer Number Mode (Next)"=IMAQdx_Buffer_Number_Mode."Last New", "Image In"=w892, "Session In"=w898) -> ("error out"=w895:errorcluster, "Image Out"=w893:T4)  [unwired: 5 in, 2 out]
                            n380 = case shown="\"No rotation, Flip LR\"" w890 {
                              tunnel: w893 -> [w907 w910 w913 w916 w923 w930 w933 w942 w949]
                              tunnel: [w907 w909 w912 w914 w919 w926 w934 w938 w945] -> w891
                              frame "No rotation, No flip", Default {
                              }
                              frame "No rotation, Flip UD" {
                                w908 = u32 0 items=["Horizontal", "Vertical", "Central", "1st Diagonal", "2nd Diagonal"] ("Type of Symmetry")
                                n381 = call "IMAQ Symmetry"("Type of Symmetry"=w908, "Image Dst"=w910, "Image Src"=w910) -> ("Image Dst Out"=w909:T4)  [unwired: 2 in, 1 out]
                              }
                              frame "No rotation, Flip LR" {
                                w911 = u32 1 items=["Horizontal", "Vertical", "Central", "1st Diagonal", "2nd Diagonal"] ("Type of Symmetry")
                                n382 = call "IMAQ Symmetry"("Type of Symmetry"=w911, "Image Dst"=w913, "Image Src"=w913) -> ("Image Dst Out"=w912:T4)  [unwired: 2 in, 1 out]
                              }
                              frame "Clockwise, No flip" {
                                n383 = call "IMAQ Rotate"("Use Bilinear Interpolation"=FALSE, "Maintain Size"=FALSE, "Angle (degrees)"=sgl 270.0, "Image Dst"=w916, "Image Src"=w916) -> ("Image Dst Out"=w914:T4)  [unwired: 5 in, 1 out]
                              }
                              frame "Clockwise, Flip UD" {
                                w921 = u32 0 items=["Horizontal", "Vertical", "Central", "1st Diagonal", "2nd Diagonal"] ("Type of Symmetry")
                                n384 = call "IMAQ Rotate"("Use Bilinear Interpolation"=FALSE, "Maintain Size"=FALSE, "Angle (degrees)"=sgl 270.0, "Image Dst"=w923, "Image Src"=w923) -> ("Image Dst Out"=w920:T4)  [unwired: 5 in, 1 out]
                                n385 = call "IMAQ Symmetry"("Type of Symmetry"=w921, "Image Dst"=w920, "Image Src"=w920) -> ("Image Dst Out"=w919:T4)  [unwired: 2 in, 1 out]
                              }
                              frame "Clockwise, Flip LR" {
                                w928 = u32 1 items=["Horizontal", "Vertical", "Central", "1st Diagonal", "2nd Diagonal"] ("Type of Symmetry")
                                n386 = call "IMAQ Rotate"("Use Bilinear Interpolation"=FALSE, "Maintain Size"=FALSE, "Angle (degrees)"=sgl 270.0, "Image Dst"=w930, "Image Src"=w930) -> ("Image Dst Out"=w927:T4)  [unwired: 5 in, 1 out]
                                n387 = call "IMAQ Symmetry"("Type of Symmetry"=w928, "Image Dst"=w927, "Image Src"=w927) -> ("Image Dst Out"=w926:T4)  [unwired: 2 in, 1 out]
                              }
                              frame "Anticlockwise, No flip" {
                                n388 = call "IMAQ Rotate"("Use Bilinear Interpolation"=FALSE, "Maintain Size"=FALSE, "Angle (degrees)"=sgl 90.0, "Image Dst"=w933, "Image Src"=w933) -> ("Image Dst Out"=w934:T4)  [unwired: 5 in, 1 out]
                              }
                              frame "Anticlockwise, Flip UD" {
                                w940 = u32 0 items=["Horizontal", "Vertical", "Central", "1st Diagonal", "2nd Diagonal"] ("Type of Symmetry")
                                n389 = call "IMAQ Rotate"("Use Bilinear Interpolation"=FALSE, "Maintain Size"=FALSE, "Angle (degrees)"=sgl 90.0, "Image Dst"=w942, "Image Src"=w942) -> ("Image Dst Out"=w939:T4)  [unwired: 5 in, 1 out]
                                n390 = call "IMAQ Symmetry"("Type of Symmetry"=w940, "Image Dst"=w939, "Image Src"=w939) -> ("Image Dst Out"=w938:T4)  [unwired: 2 in, 1 out]
                              }
                              frame "Anticlockwise, Flip LR" {
                                w947 = u32 1 items=["Horizontal", "Vertical", "Central", "1st Diagonal", "2nd Diagonal"] ("Type of Symmetry")
                                n391 = call "IMAQ Rotate"("Use Bilinear Interpolation"=FALSE, "Maintain Size"=FALSE, "Angle (degrees)"=sgl 90.0, "Image Dst"=w949, "Image Src"=w949) -> ("Image Dst Out"=w946:T4)  [unwired: 5 in, 1 out]
                                n392 = call "IMAQ Symmetry"("Type of Symmetry"=w947, "Image Dst"=w946, "Image Src"=w946) -> ("Image Dst Out"=w945:T4)  [unwired: 2 in, 1 out]
                              }
                            }
                            n393 = case shown="False" w906 {
                              tunnel: w905 -> [w989 _]
                              tunnel: w897 -> [w990 _]
                              tunnel: w891 -> [w988 _]
                              tunnel: w899 -> [w987 _]
                              frame False {
                                n394 = case shown="3" w990 {
                                selector: w990 -> [_ w991]
                                tunnel: w989 -> [_ w995]
                                tunnel: w988 -> [_ w994]
                                tunnel: w987 -> [_ w993]
                                frame -1, Default {
                                }
                                frame 3 {
                                n395 = call "IMAQ Copy"("Image Dst"=w995, "Image Src"=w994) -> ("Image Dst Out"=w992:T4)  [unwired: 4 in, 1 out]
                                n396 = case shown="3" w991 {
                                tunnel: w993 -> [_ w997]
                                tunnel: w992 -> [_ w996]
                                frame 0, Default {
                                }
                                frame 3 {
                                n397 = property class="ImageControl"(reference=w997, "Value"=w996) -> ()  [unwired: 1 in, 2 out]
                                }
                                }
                                }
                                }
                              }
                              frame True {
                              }
                            }
                            n398 = case shown="\"dat\", \"u16\"" w902 {
                              tunnel: w891 -> [w959 _ w979]
                              tunnel: w903 -> [_ _ w978]
                              tunnel: w901 -> [w956 _ _]
                              tunnel: w900 -> [w957 _ _]
                              tunnel: w894 -> [w955 _ _]
                              tunnel: w889 -> [w954 _ w977]
                              tunnel: w896 -> [w953 _ w974]
                              tunnel: w895 -> [w952 _ w976]
                              frame "'tiff'", "tif" {
                                n399 = in-place {
                                in-place-border: w959 -> [w973]
                                in-place-border: w952 -> [w972]
                                n400 = in-place-dvr #4(w957) -> ()  [unwired: 2 out]
                                n401 = call "IMAQ ImageToArray"("error in (no error)"=w972, "Image"=w973) -> ("Image Pixels (I16)"=w971:i16[][])  [unwired: 2 in, 4 out]
                                n402 = in-place-dvr #4(w971) -> (w958:refnum<data-value>)  [unwired: 1 out]
                                }
                                n403 = stacked-sequence {
                                tunnel: w958 -> [_ w967 _ _]
                                tunnel: w956 -> [_ w966 _ _]
                                tunnel: w955 -> [_ w965 _ _]
                                tunnel: w954 -> [w960 _ _ w970]
                                tunnel: w953 -> [_ _ w969 _]
                                frame #0 {
                                n404 = call <vilib>:"Acquire Semaphore.vi"("semaphore"=w960) -> ()  [unwired: 4 in, 3 out]
                                }
                                frame #1 {
                                n405 = Preview Queue Element(queue=w965) -> (queue out=w963:refnum<queue>, element=w964:u32[])  [unwired: 2 in, 2 out]
                                n406 = call "TIFFStream Write.vi"("File data"=w966, "Last image in file?"=FALSE, "Current and next IFD offset in"=w964, "Image data reference"=w967) -> ("Current and next IFD offset out"=w962:u32[])  [unwired: 6 in, 1 out]
                                n407 = Lossy Enqueue Element(queue=w963, element=w962) -> ()  [unwired: 1 in, 4 out]
                                }
                                frame #2 {
                                n408 = Enqueue Element(queue=w969, element=enum16{"Camera 1", "Camera 2", "Camera 3"}."Camera 3") -> ()  [unwired: 2 in, 3 out]
                                }
                                frame #3 {
                                n409 = call <vilib>:"Release Semaphore.vi"("semaphore"=w970) -> ()  [unwired: 5 in, 2 out]
                                }
                                }
                              }
                              frame "None", Default {
                              }
                              frame "dat", "u16" {
                                n410 = call "IMAQ ImageToArray"("error in (no error)"=w976, "Image"=w979) -> ("Image Pixels (I16)"=w975:i16[][])  [unwired: 2 in, 4 out]
                                n411 = stacked-sequence {
                                tunnel: w975 -> [_ w982 _ _]
                                tunnel: w978 -> [_ w981 _ _]
                                tunnel: w977 -> [w980 _ _ w986]
                                tunnel: w974 -> [_ _ w984 _]
                                frame #0 {
                                n412 = call <vilib>:"Acquire Semaphore.vi"("semaphore"=w980) -> ()  [unwired: 4 in, 3 out]
                                }
                                frame #1 {
                                n413 = Write to Binary File(file (use dialog)=w981, data=w982, 5:FALSE ("prepend array or string size? (T)")) -> ()  [unwired: 3 in, 3 out]
                                }
                                frame #2 {
                                n414 = Enqueue Element(queue=w984, element=enum16{"Camera 1", "Camera 2", "Camera 3"}."Camera 3") -> ()  [unwired: 2 in, 3 out]
                                }
                                frame #3 {
                                n415 = call <vilib>:"Release Semaphore.vi"("semaphore"=w986) -> ()  [unwired: 5 in, 2 out]
                                }
                                }
                              }
                            }
                            n416 = property class="Bool (strict)"(reference=w888) -> ("Value"=w887:bool)  [unwired: 1 in, 2 out]
                            n417 = Not(x=w887) -> (.not. x?=w886:bool)
                          }
                        }
                      }
                    }
                    frame True {
                    }
                  }
                }
                frame #1 {
                  n418 = Send Notification(notification=TRUE, notifier=w1299) -> ()  [unwired: 1 in, 2 out]
                }
              }
              n419 = node-c288(i64 33 ("Period"), 10 ("Priority")) -> (w723:T13)  [unwired: 2 in]
              n420 = timed-loop {
                timing: w723 -> [_]
                timing-out: [_] -> w722
                tunnel: w721 -> [w745]
                tunnel: w718 -> [w740]
                tunnel: w717 -> [w743]
                tunnel: w714 -> [w738]
                tunnel: w713 -> [_]
                stop <- w744 stop-if-true
                n421 = node-c288() -> ()  [unwired: 1 in, 1 out]
                n422 = Get Notifier Status(notifier=w745) -> (current notification=w744:bool)  [unwired: 1 in, 4 out]
                n423 = Unbundle By Name(w743) -> ("Offset and gain"=w742:dbl[][], "RGB Channels"=w741:T19, "RGB buffers"=w739:T4[], "Current camera"=w737:i32)
                n424 = case shown="0" w737 {
                  tunnel: w742 -> [_ w767]
                  tunnel: w741 -> [_ w766]
                  tunnel: w740 -> [_ w765]
                  tunnel: w739 -> [_ w763]
                  tunnel: w738 -> [_ w760]
                  frame 1, Default {
                  }
                  frame 0 {
                    w751 = u16 0 items=["RGB", "HSL", "HSV", "HSI"] ("Color Mode")
                    n425 = Index Array(array=w763, index #1=0 ("index"), index #2=1 ("index")) -> (element #1=w761:T4, element #2=w758:T4)
                    n426 = Array Subset(array=w763, index=2 ("length"), length=3 ("index")) -> (w764:T4[])
                    n427 = for {
                      tunnel: w764 -> [w773] mode=indexing
                      tunnel: w767 -> [w772] mode=indexing
                      tunnel: w766 -> [w775] mode=indexing
                      tunnel: w765 -> [w774]
                      tunnel: [w771] -> w757 mode=indexing
                      tunnel: w758 -> [w770]
                      n428 = case shown="\"Camera 1\", Default" w775 {
                        selector: w775 -> [_ w796]
                        tunnel: w774 -> [_ w795]
                        tunnel: w773 -> [w778 w780]
                        tunnel: w772 -> [_ w790]
                        tunnel: [w776 w779] -> w771
                        tunnel: w770 -> [_ w792]
                        frame "None" {
                          n429 = call "IMAQ FillImage"("Pixel Value (U8, U16, I16, Float)"=sgl 0.0, "Image"=w778) -> ("Image Out"=w776:T4)  [unwired: 8 in, 1 out]
                        }
                        frame "Camera 1", Default {
                          w781 = T18 0 items=["Grayscale (U8)", "Grayscale (I16)", "Grayscale (SGL)", "Complex (CSG)", "RGB (U32)", "HSL (U32)", "RGB (U64)", "Grayscale (U16)"] ("Image Type")
                          w791 = T18 2 items=["Grayscale (U8)", "Grayscale (I16)", "Grayscale (SGL)", "Complex (CSG)", "RGB (U32)", "HSL (U32)", "RGB (U64)", "Grayscale (U16)"] ("Image Type")
                          n430 = Decrement(x=w796) -> (x-1=w794:T21)
                          n431 = Index Array(array=w795, index=w794) -> (element=w793:T4)
                          n432 = Index Array(array=w790, index #1=0 ("index"), index #2=1 ("index")) -> (element #1=w787:dbl, element #2=w783:dbl)
                          n433 = call "IMAQ Cast Image"("Image Type"=w791, "Image Dst"=w792, "Image Src"=w793) -> ("Image Dst Out"=w786:T4)  [unwired: 7 in, 1 out]
                          n434 = call "IMAQ Add"("Image Src A"=w786, "Constant"=w787, "Image Dst"=w786) -> ("Image Dst Out"=w784:T4, "error out"=w785:errorcluster)  [unwired: 4 in]
                          n435 = call "IMAQ Multiply"("Image Src A"=w784, "Constant"=w783, "Image Dst"=w784, "error in (no error)"=w785) -> ("Image Dst Out"=w782:T4)  [unwired: 3 in, 1 out]
                          n436 = call "IMAQ Cast Image"("Image Type"=w781, "Image Dst"=w780, "Image Src"=w782) -> ("Image Dst Out"=w779:T4)  [unwired: 7 in, 1 out]
                        }
                      }
                    }
                    n437 = Index Array(array=w757, index #1=0 ("index"), index #2=1 ("index"), index #3=2 ("index")) -> (element #1=w748:T4, element #2=w753:T4, element #3=w752:T4)
                    n438 = call "IMAQ GetImageSize"("Image"=w748) -> ("Y Resolution"=w746:i32, "X Resolution"=w747:i32)  [unwired: 3 in, 1 out]
                    n439 = call "IMAQ SetImageSize"("Y Resolution"=w746, "X Resolution"=w747, "Image"=w761) -> ("Image Out"=w749:T4)  [unwired: 2 in, 1 out]
                    n440 = call "IMAQ ReplaceColorPlane"("Image Src"=w749, "Color Mode"=w751, "Image Dst"=w749, "Red or Hue Plane"=w748, "Green or Sat Plane"=w753, "Blue or Luma or Val or Inten Plane"=w752) -> ("Image Dst Out"=w750:T4)  [unwired: 8 in, 1 out]
                    n441 = property class="ImageControl"(reference=w760, "Value"=w750) -> ()  [unwired: 1 in, 2 out]
                  }
                }
                n442 = node-c288() -> ()  [unwired: 1 in, 1 out]
              }
              n443 = node-c288(w722) -> ()  [unwired: 1 out]
            }
            frame #3 {
              n444 = disable-structure shown="Enabled" {
                disable-tunnel: w1307 -> [_ w1349]
                frame Disabled {
                }
                frame Enabled {
                  n445 = for {
                    tunnel: w1349 -> [w1351] mode=indexing
                    n446 = call <vilib>:"IMAQdx Stop Acquisition.vi"("Session In"=w1351) -> ("Session Out"=w1350:T3)  [unwired: 9 in, 1 out]
                    n447 = call <vilib>:"IMAQdx Unconfigure Acquisition.vi"("Session In"=w1350) -> ()  [unwired: 9 in, 2 out]
                  }
                }
              }
              n448 = case shown="\"dat\", \"u16\"" w1306 {
                tunnel: w1305 -> [_ _ w1343]
                tunnel: w1304 -> [w1324 _ _]
                tunnel: w1303 -> [w1323 _ _]
                tunnel: w1302 -> [w1311 _ w1335]
                tunnel: w1301 -> [w1318 _ w1342]
                tunnel: w1300 -> [w1317 _ _]
                frame "'tiff'", "tif" {
                  n449 = Flush Queue(queue=w1311) -> (queue out=w1315:refnum<queue>, remaining elements=w1314:enum16{"Camera 1", "Camera 2", "Camera 3"}[], error out=w1313:errorcluster)  [unwired: 1 in]
                  n450 = Preview Queue Element(queue=w1317) -> (element=w1316:u32[])  [unwired: 2 in, 3 out]
                  n451 = call "TIFFStream Close.vi"("Current and next IFD offset"=w1316, "Image data reference"=w1323, "File data"=w1324) -> ()  [unwired: 8 in, 1 out]
                  n452 = for {
                    tunnel: w1314 -> [w1326] mode=indexing
                    tunnel: [w1325] -> w1312 mode=indexing
                    n453 = case shown="\"Camera 1\", Default" w1326 {
                      tunnel: ["1" "2" "3"] -> w1325
                      frame "Camera 1", Default {
                      }
                      frame "Camera 2" {
                      }
                      frame "Camera 3" {
                      }
                    }
                  }
                  n454 = Release Queue(queue=w1315, error in (no error)=w1313) -> ()  [unwired: 1 in, 3 out]
                  n455 = Strip Path(path=w1318) -> (stripped path=w1322:path)  [unwired: 1 out]
                  n456 = call <vilib>:"Get File Extension.vi"("file"=w1318) -> ("filename without extension"=w1320:string)  [unwired: 6 in, 4 out]
                  n457 = Concatenate Strings(w1320, "_FrameOrder.txt" ("string")) -> (w1321:string)
                  n458 = Build Path(base path=w1322, name or relative path=w1321) -> (appended path=w1310:path)
                  n459 = Concatenate Strings(w1312) -> (w1309:string)
                  n460 = Write to Text File(file (use dialog)=w1310, text=w1309) -> (refnum out=w1308:refnum<file>)  [unwired: 2 in, 2 out]
                  n461 = Close File(refnum=w1308) -> ()  [unwired: 1 in, 2 out]
                }
                frame "None", Default {
                }
                frame "dat", "u16" {
                  n462 = Close File(refnum=w1343) -> ()  [unwired: 1 in, 2 out]
                  n463 = Flush Queue(queue=w1335) -> (queue out=w1336:refnum<queue>, remaining elements=w1334:enum16{"Camera 1", "Camera 2", "Camera 3"}[], error out=w1333:errorcluster)  [unwired: 1 in]
                  n464 = Strip Path(path=w1342) -> (stripped path=w1341:path)  [unwired: 1 out]
                  n465 = call <vilib>:"Get File Extension.vi"("file"=w1342) -> ("filename without extension"=w1339:string)  [unwired: 6 in, 4 out]
                  n466 = for {
                    tunnel: w1334 -> [w1345] mode=indexing
                    tunnel: [w1344] -> w1332 mode=indexing
                    n467 = case shown="\"Camera 1\", Default" w1345 {
                      tunnel: ["1" "2" "3"] -> w1344
                      frame "Camera 1", Default {
                      }
                      frame "Camera 2" {
                      }
                      frame "Camera 3" {
                      }
                    }
                  }
                  n468 = Concatenate Strings(w1339, "_FrameOrder.txt" ("string")) -> (w1340:string)
                  n469 = Release Queue(queue=w1336, error in (no error)=w1333) -> ()  [unwired: 1 in, 3 out]
                  n470 = Build Path(base path=w1341, name or relative path=w1340) -> (appended path=w1337:path)
                  n471 = Concatenate Strings(w1332) -> (w1331:string)
                  n472 = Write to Text File(file (use dialog)=w1337, text=w1331) -> (refnum out=w1330:refnum<file>)  [unwired: 2 in, 2 out]
                  n473 = Close File(refnum=w1330) -> ()  [unwired: 1 in, 2 out]
                }
              }
            }
          }
        }
      }
    }
    frame "Get status" {
      n474 = Variant To Data(type=w1361, Variant=w1362) -> (data=w1360:T6)  [unwired: 1 in, 1 out]
      n475 = Unbundle By Name(w1360) -> ("Camera References"=w1359:T3[], "Current camera"=w1358:i32)
      n476 = Decrement(x=w1358) -> (x-1=w1354:i32)
      n477 = Max & Min(x=w1354, y=1) -> (max(x,y)=w1352:i32)  [unwired: 1 out]
      n478 = Index Array(array=w1359, index=w1352) -> (element=w1357:T3)
      n479 = property class="IMAQdx"(reference=w1357, "ActiveAttribute"="CameraAttributes::DeviceControl::DeviceTemperature") -> (error out=w1356:errorcluster, "ValueDBL"=w1363:dbl)  [unwired: 1 in, 1 out]
      n480 = Unbundle By Name(w1356) -> ("status"=w1355:bool)
      n481 = Bundle By Name(cluster=w1366, "System OK?"=w1355, "Temperature"=w1363) -> (w1365:T1)
    }
    frame "Other settings" {
      n482 = Variant To Data(type=w1382, Variant=w1383) -> (data=w1378:T6)  [unwired: 1 in, 1 out]
      n483 = Unbundle By Name(w1378) -> ("Offset and gain"=w1369:dbl[][], "Camera References"=w1381:T3[], "Current camera"=w1380:i32, "Which cameras record"=w1379:bool[], "RGB Channels"=w1371:T19, "Image buffers"=w1370:T4[], "Camera orientation"=w1368:T17)
      n484 = call "PointGrey Grasshopper_Settings.vi"("Camera References"=w1381, "Offset and gain"=w1369, "Camera to address"=w1380, "Camera orientation"=w1368, "Which cameras record"=w1379, "RGB Channels in"=w1371, "Image buffers"=w1370) -> ("Offset gain out"=w1373:dbl[][], "Camera to address out"=w1374:i32, "Camera orientation out"=w1367:T17, "Which cameras record out"=w1377:bool[], "RGB Channels out"=w1372:T19)  [unwired: 4 in]
      n485 = Bundle By Name(cluster=w1378, "Offset and gain"=w1373, "Current camera"=w1374, "Which cameras record"=w1377, "RGB Channels"=w1372, "Camera orientation"=w1367) -> (w1375:T6)
      n486 = To Variant(anything=w1375) -> (Variant=w1376:variant)
    }
  }
  "Status" <- w8
  "Camera-specific out" <- w5
